vi "cDAQ_VI_Leo_Autotuning.vi"() -> ()   [LabVIEW 2022 SP3]
uses:
  <vilib>/addons/control/pid/autopid.llb/PID autotuning parameters.ctl
  <vilib>/Analysis/baseanly.llb/Mean (DBL).vi
  <vilib>/DAQmx/read.llb/DAQmx Read (Analog 1D Wfm NChan NSamp).vi
  STOP_GLOBAL.vi
  <vilib>/DAQmx/configure/timing.llb/DAQmx Timing (Sample Clock).vi
  <vilib>/addons/control/pid/pid.llb/PID Lead-Lag (DBL).vi
  <vilib>/addons/control/pid/pid.llb/PID Gain Schedule (DBL).vi
  <vilib>/addons/control/pid/pid.llb/PID (DBL).vi
  <vilib>/DAQmx/miscellaneous.llb/DAQmx Fill In Error Info.vi
  <vilib>/Analysis/NI_AALBase.lvlib
  <vilib>/addons/control/pid/NI_PID_pid.lvlib
  <vilib>/ptbypt/NI_PtbyPt.lvlib
  <resource>/objmgr/daqmx.rc
panel:
  out "Inlet Pressure":dynamicdata(graph)
  in  "Channel Array":dbl[](array[slide]) scale=0.0..5.067
  in  "Pressure Scheduling":T1(array[cluster])=[{"PID gains"={"Kc"=7.0, "Ti"=0.001, "Td"=0.0}, "max value"=0.0}] {"max value" format="%.2f"; "PID gains"."Td" format="%#.3g"; "PID gains"."Ti" format="%#.3g"; "PID gains"."Kc" format="%#.3g"}
  out "Runtime Passed?":bool
  in  "RunTime":dbl
  out "Entire Runtime":dbl
  out "Actual Clock Rate":dbl
  out "error out 4":errorcluster
  out "Setpoint profile":dbl
  out "Second Pressure Transducer":cluster{dbl[], dbl[]}(graph)
  out "Second Pressure Transducer":dynamicdata(graph)
  out "Servo Voltage Output":cluster{dbl[], dbl[]}(graph)
  in  "Tab Control":T2(tab)
  out "error out 5":errorcluster
  in  "stop":bool
  in  "Needle Valve Control":dbl[](array[slide]) scale=0.0..1.0
  out "Waveform Chart":cluster{"SP":dbl, dbl}(graph)
  out "Output":dbl(slide) scale=0.0..5.067
  out "Process Variable vs Setpoint":cluster{dbl[], dbl[]}[](graph)
  out "error out":errorcluster
  out "element":dbl
  out "MVT Process variable":dbl
  out "MVT Setpoint":dbl
  in  "SP":dbl format="%.2f"
  out "PID gains out":T3={"proportional gain (Kc)"=1.0, "integral time (Ti, min)"=0.01, "derivative time (Td, min)"=0.0} {"derivative time (Td, min)" format="%.3f"; "integral time (Ti, min)" format="%.3f"; "proportional gain (Kc)" format="%.3f"}
  in  "Insert Gain":bool
  out "output":dbl format="%.2f"
  in  "Autotune":bool
  in  "Reinitialize":bool
  in  "Automatic":bool=TRUE
  in  "Replace Gain":bool
  in  "alpha":dbl=nan format="%.2f"
  out "tuned PID gains":T3={"proportional gain (Kc)"=1.0, "integral time (Ti, min)"=0.01, "derivative time (Td, min)"=0.0} {"derivative time (Td, min)" format="%.3f"; "integral time (Ti, min)" format="%.3f"; "proportional gain (Kc)" format="%.3f"}
  out "Voltage Output":dynamicdata(graph)
  in  "autotuning parameters":T4={"type of controller"=0, "relay cycles"=3, "relay amplitude"=1.0, "control specifications"=2, "PV noise level"=0.1} {"PV noise level" format="%.2f"; "control specifications" items=["normal", "fast", "slow"]; "relay amplitude" format="%.2f"; "type of controller" items=["P", "PI", "PID"]}
  out "index out":i32
  in  "MV:":dbl(slide)=30.8641975308642 scale=0.0..5.067 scale format="%.1f"
  out "Waiting \nfor Start":bool=TRUE
  in  "Start VI":bool
  out "Time":dbl
  in  "Gain Schedule":T1(array[cluster])=[{"PID gains"={"Kc"=7.0, "Ti"=0.001, "Td"=0.0}, "max value"=0.0}] {"max value" format="%.2f"; "PID gains"."Td" format="%#.3g"; "PID gains"."Ti" format="%#.3g"; "PID gains"."Kc" format="%#.3g"}
  out "Steps on Servo":dbl[](array[numeric])
  out "Elapsed Time (s) 2":dbl caption="Elapsed Time (s)"
  out "HAS 3 SECONDS PASSED?":bool
  in  "PRESS TO START":bool
  out "All Channel Graph":cluster{dbl[], dbl[]}[](graph)
  out "Thrust":cluster{dbl[], dbl[]}(graph)
  out "Chamber Pressure":cluster{dbl[], dbl[]}(graph)
  out "Supply Pressure":cluster{dbl[], dbl[]}(graph)
  out "MassFlow":cluster{dbl[], dbl[]}(graph)
  out "Temperature":cluster{dbl[], dbl[]}(graph)
  out "error out 3":errorcluster caption="error out"
  out "error out 2":errorcluster
  in  "rate":dbl=1000.0 format="%0.2f"
  in  "number of samples":i32=100
  in  "File Format":string
  in  "File Name Out":string
  in  "Data Collection Folder":path
  out "Temperature":dynamicdata(graph)
  out "Thrust lb":dynamicdata(graph)
  in  "Types of Testing":enum32{"Test Firing", "Cold Flow Rig"}(tab)
  out "Saving Data":bool
  out "Filename Out":path
  in  "Collect Data?":bool=TRUE caption="Enable"
  in  "Collect Data? 2":bool=TRUE caption="Enable"
  out "Saving Data":bool
  out "Filename Out":path
  out "Supply Pressure PSI":dynamicdata(graph)
  out "Vol Flow L/min":dynamicdata(graph)
  out "Chamber Pressure PSI":dynamicdata(graph)
  # "DATA LOGGING INFORMATION"
  # "Control Loop"
  # "ANALOG VOLTAGE OUTPUT"
  # "RESULTS"
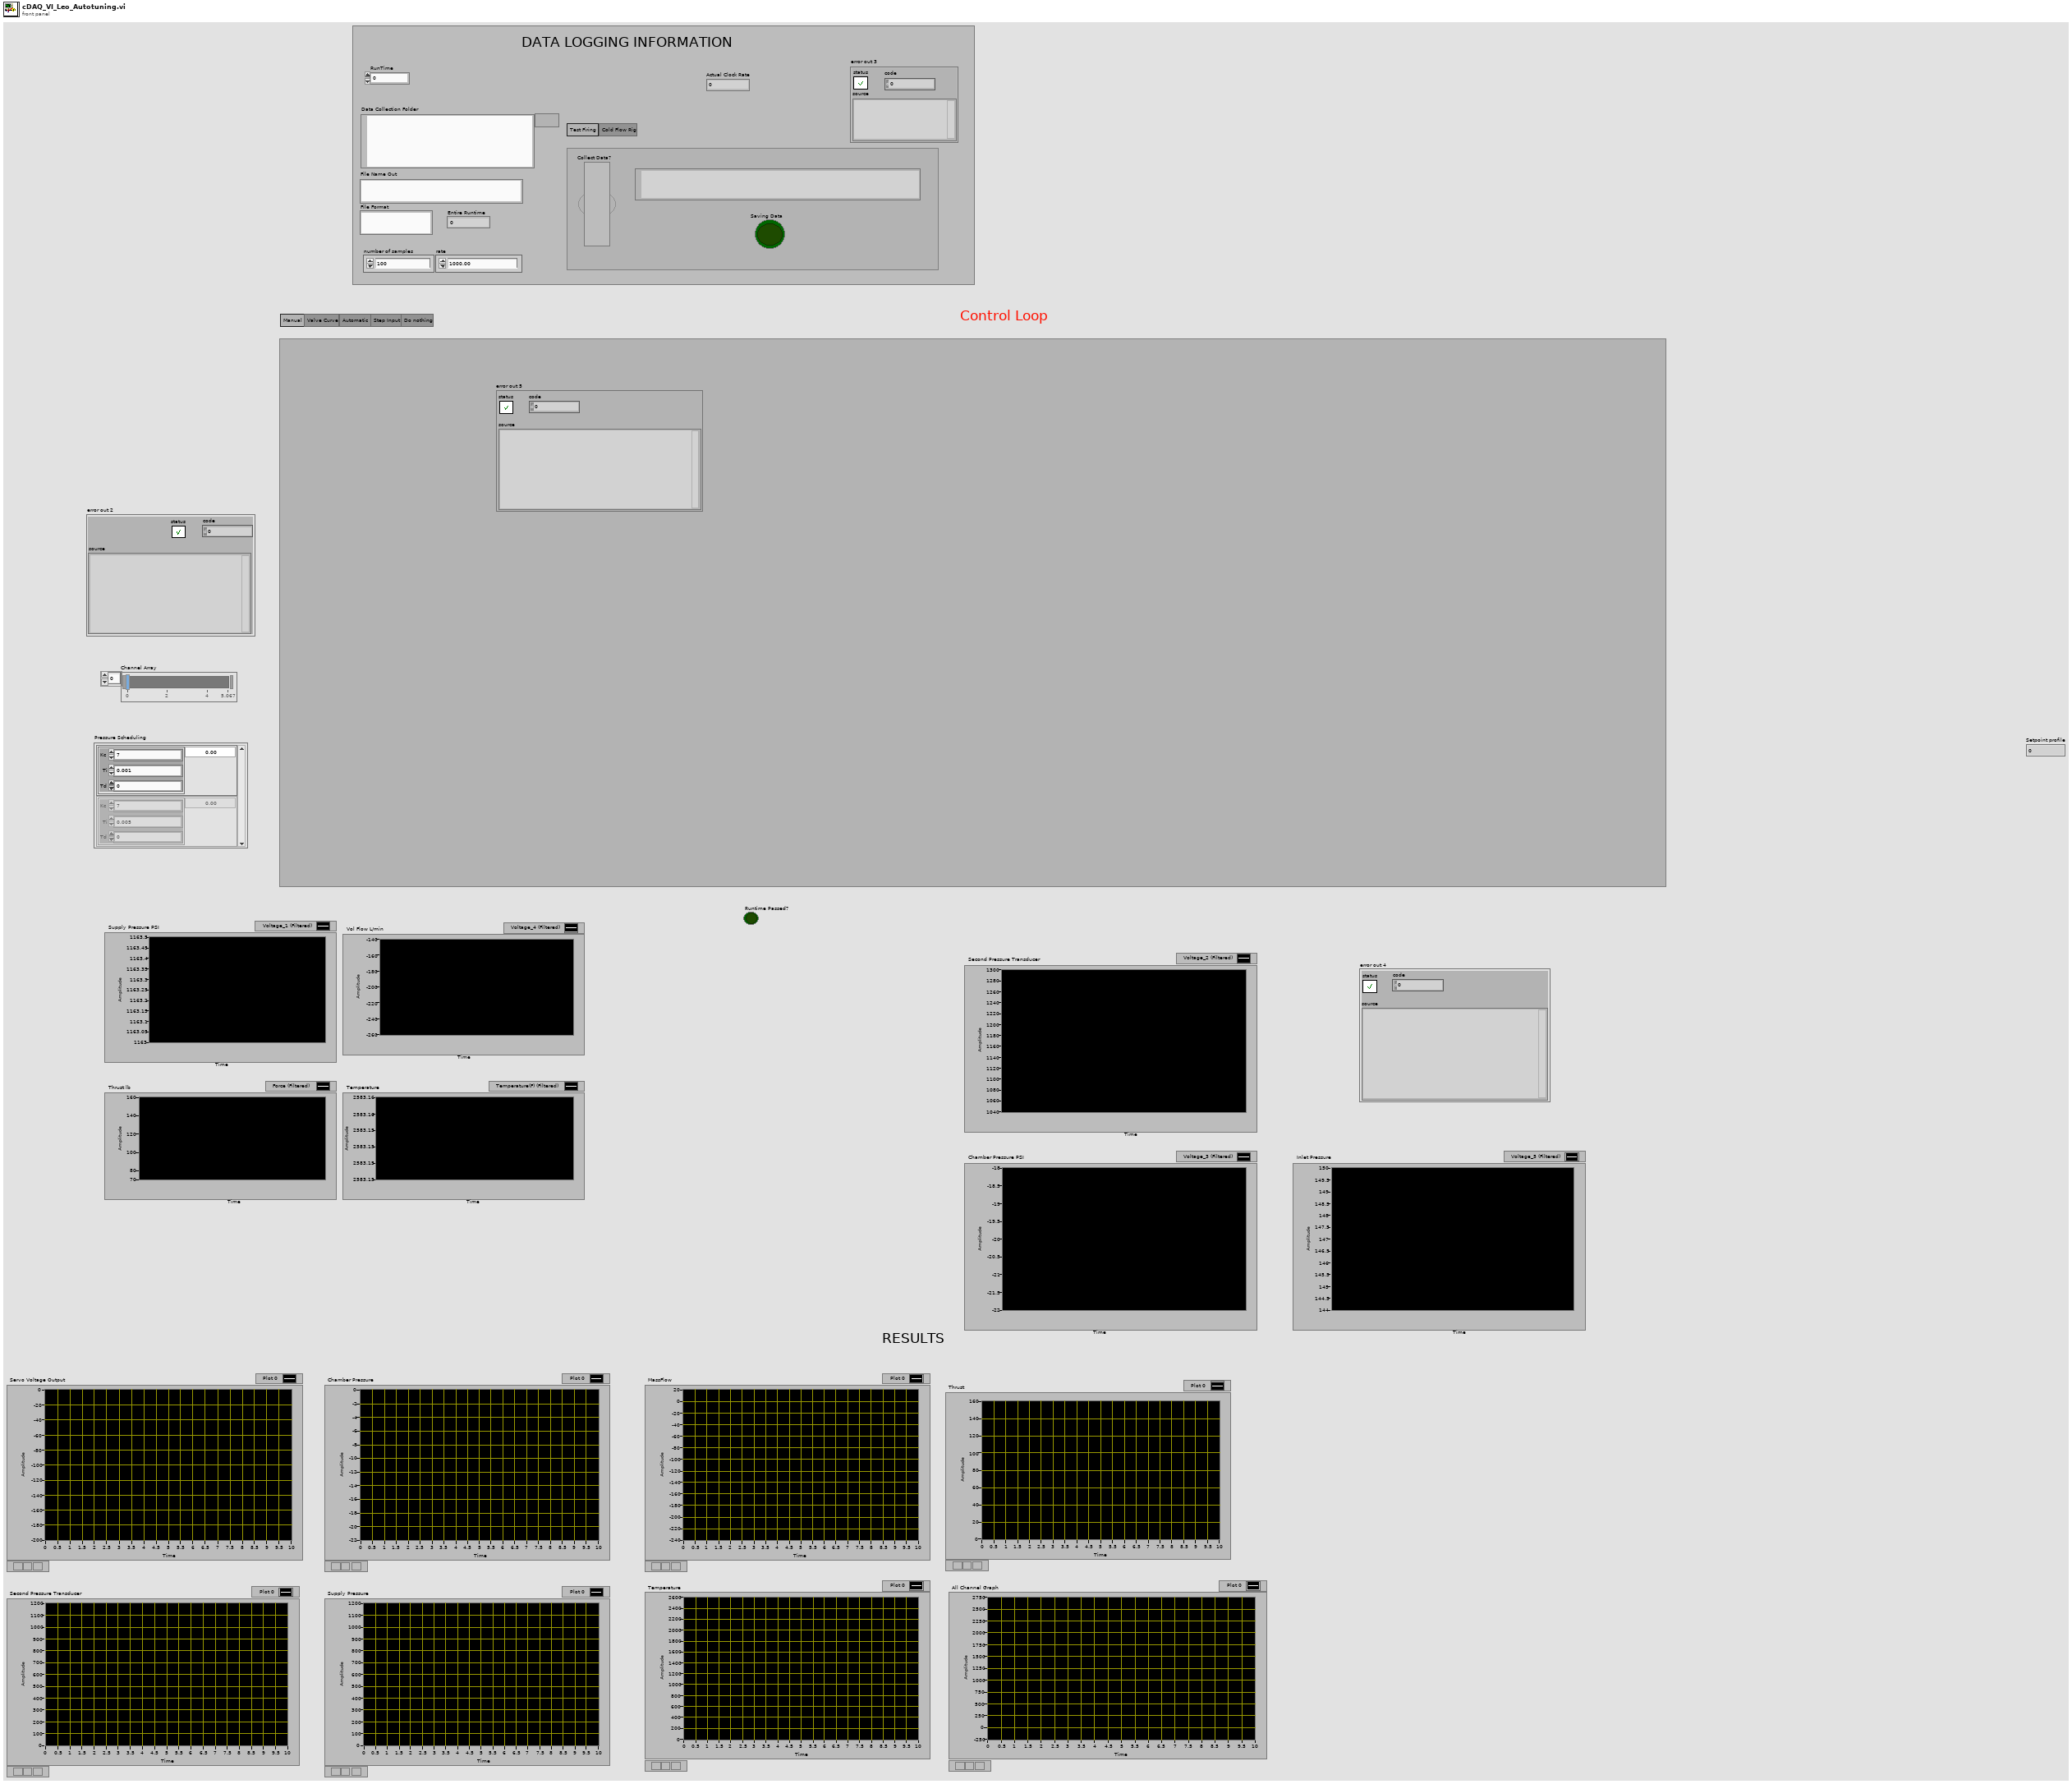
[diagram p1: front panel]
types:
  T1 = cluster{"PID gains":cluster{"Kc":dbl, "Ti":dbl, "Td":dbl}, "max value":dbl}[]
  T2 = enum32{"Manual", "Valve Curve", "Automatic", "Step Input", "Do nothing"}
  T3 = cluster{"proportional gain (Kc)":dbl, "integral time (Ti, min)":dbl, "derivative time (Td, min)":dbl}
  T4 = typedef "PID autotuning parameters.ctl" = cluster{"type of controller":u16, "relay cycles":i32, "relay amplitude":dbl, "control specifications":u16, "PV noise level":dbl}
  T5 = cluster{"Modulus":dbl, "Number of\nComplete Cycles":dbl}
  T6 = cluster{"PID gains":cluster{"Kc":dbl, "Ti":dbl, "Td":dbl}, "max value":dbl}
  T7 = cluster{"Tuned PID gains":cluster{"proportional gain (Kc)":dbl, "integral time (Ti, min)":dbl, "derivative time (Td, min)":dbl}, "MVT Process Variable":dbl}
  T8 = cluster{"Tuned PID gains":cluster{"proportional gain (Kc)":dbl, "integral time (Ti, min)":dbl, "derivative time (Td, min)":dbl}, "max value":dbl}
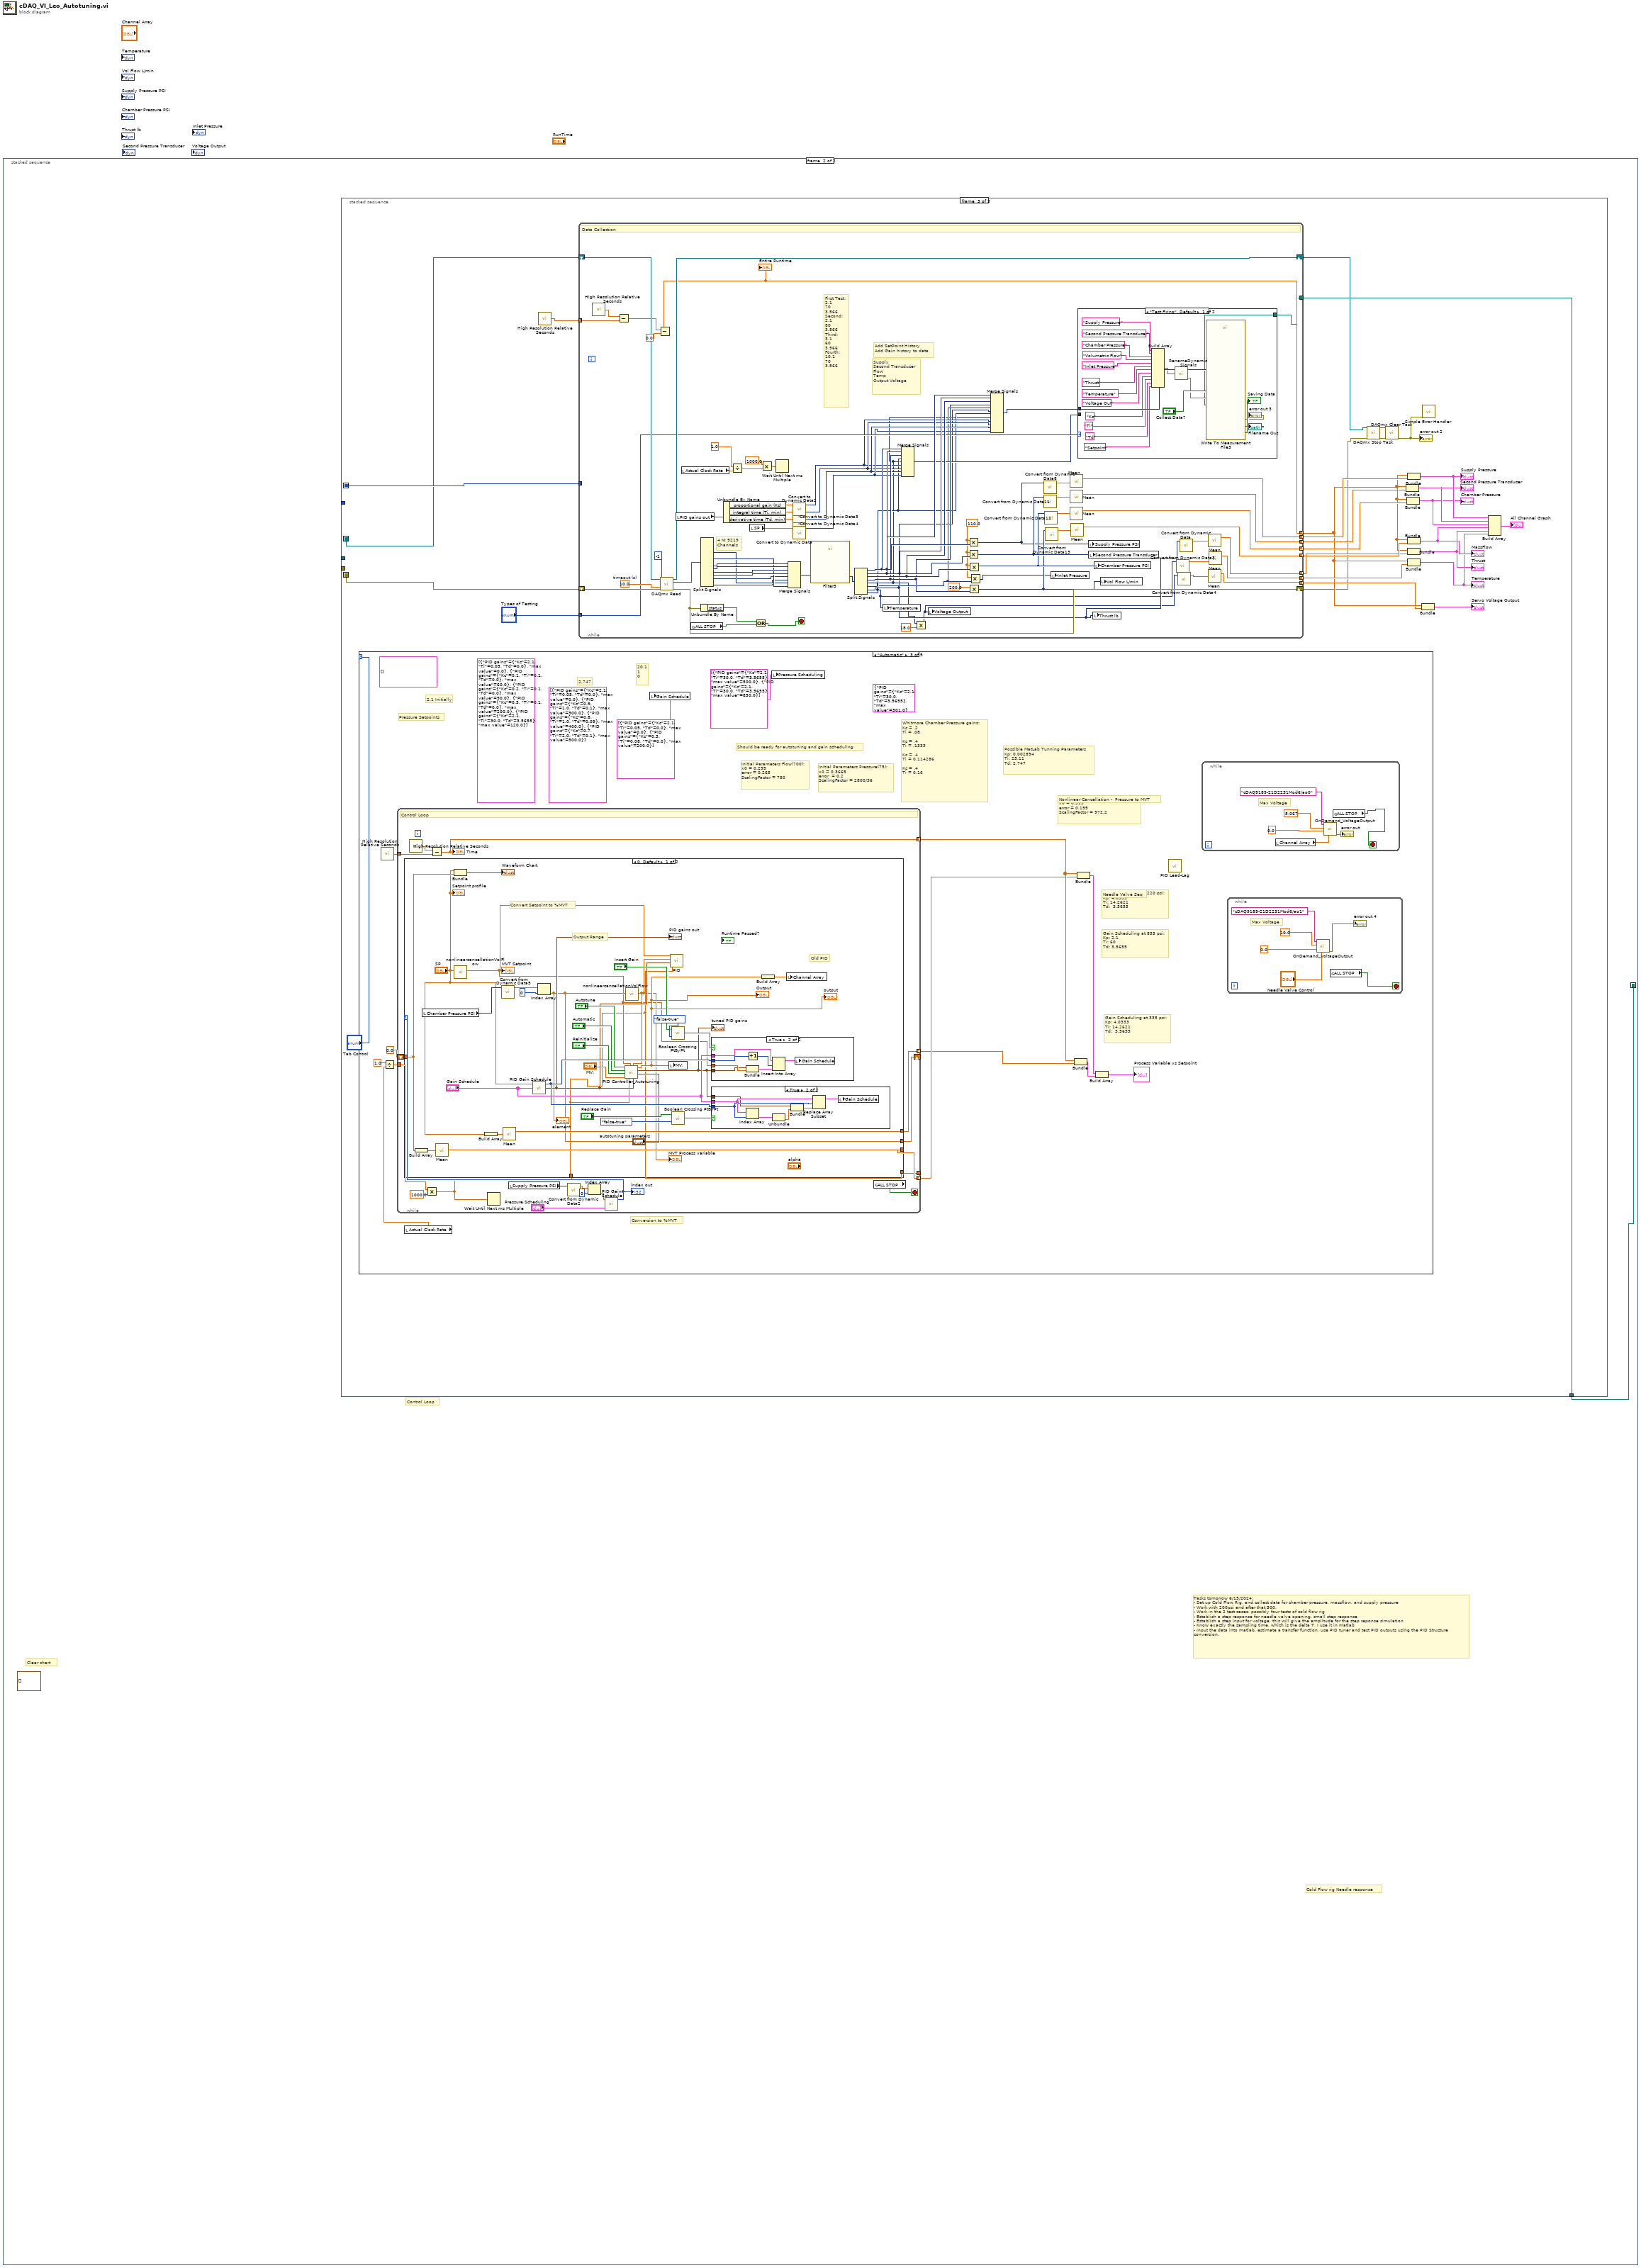
[diagram p0: block diagram]
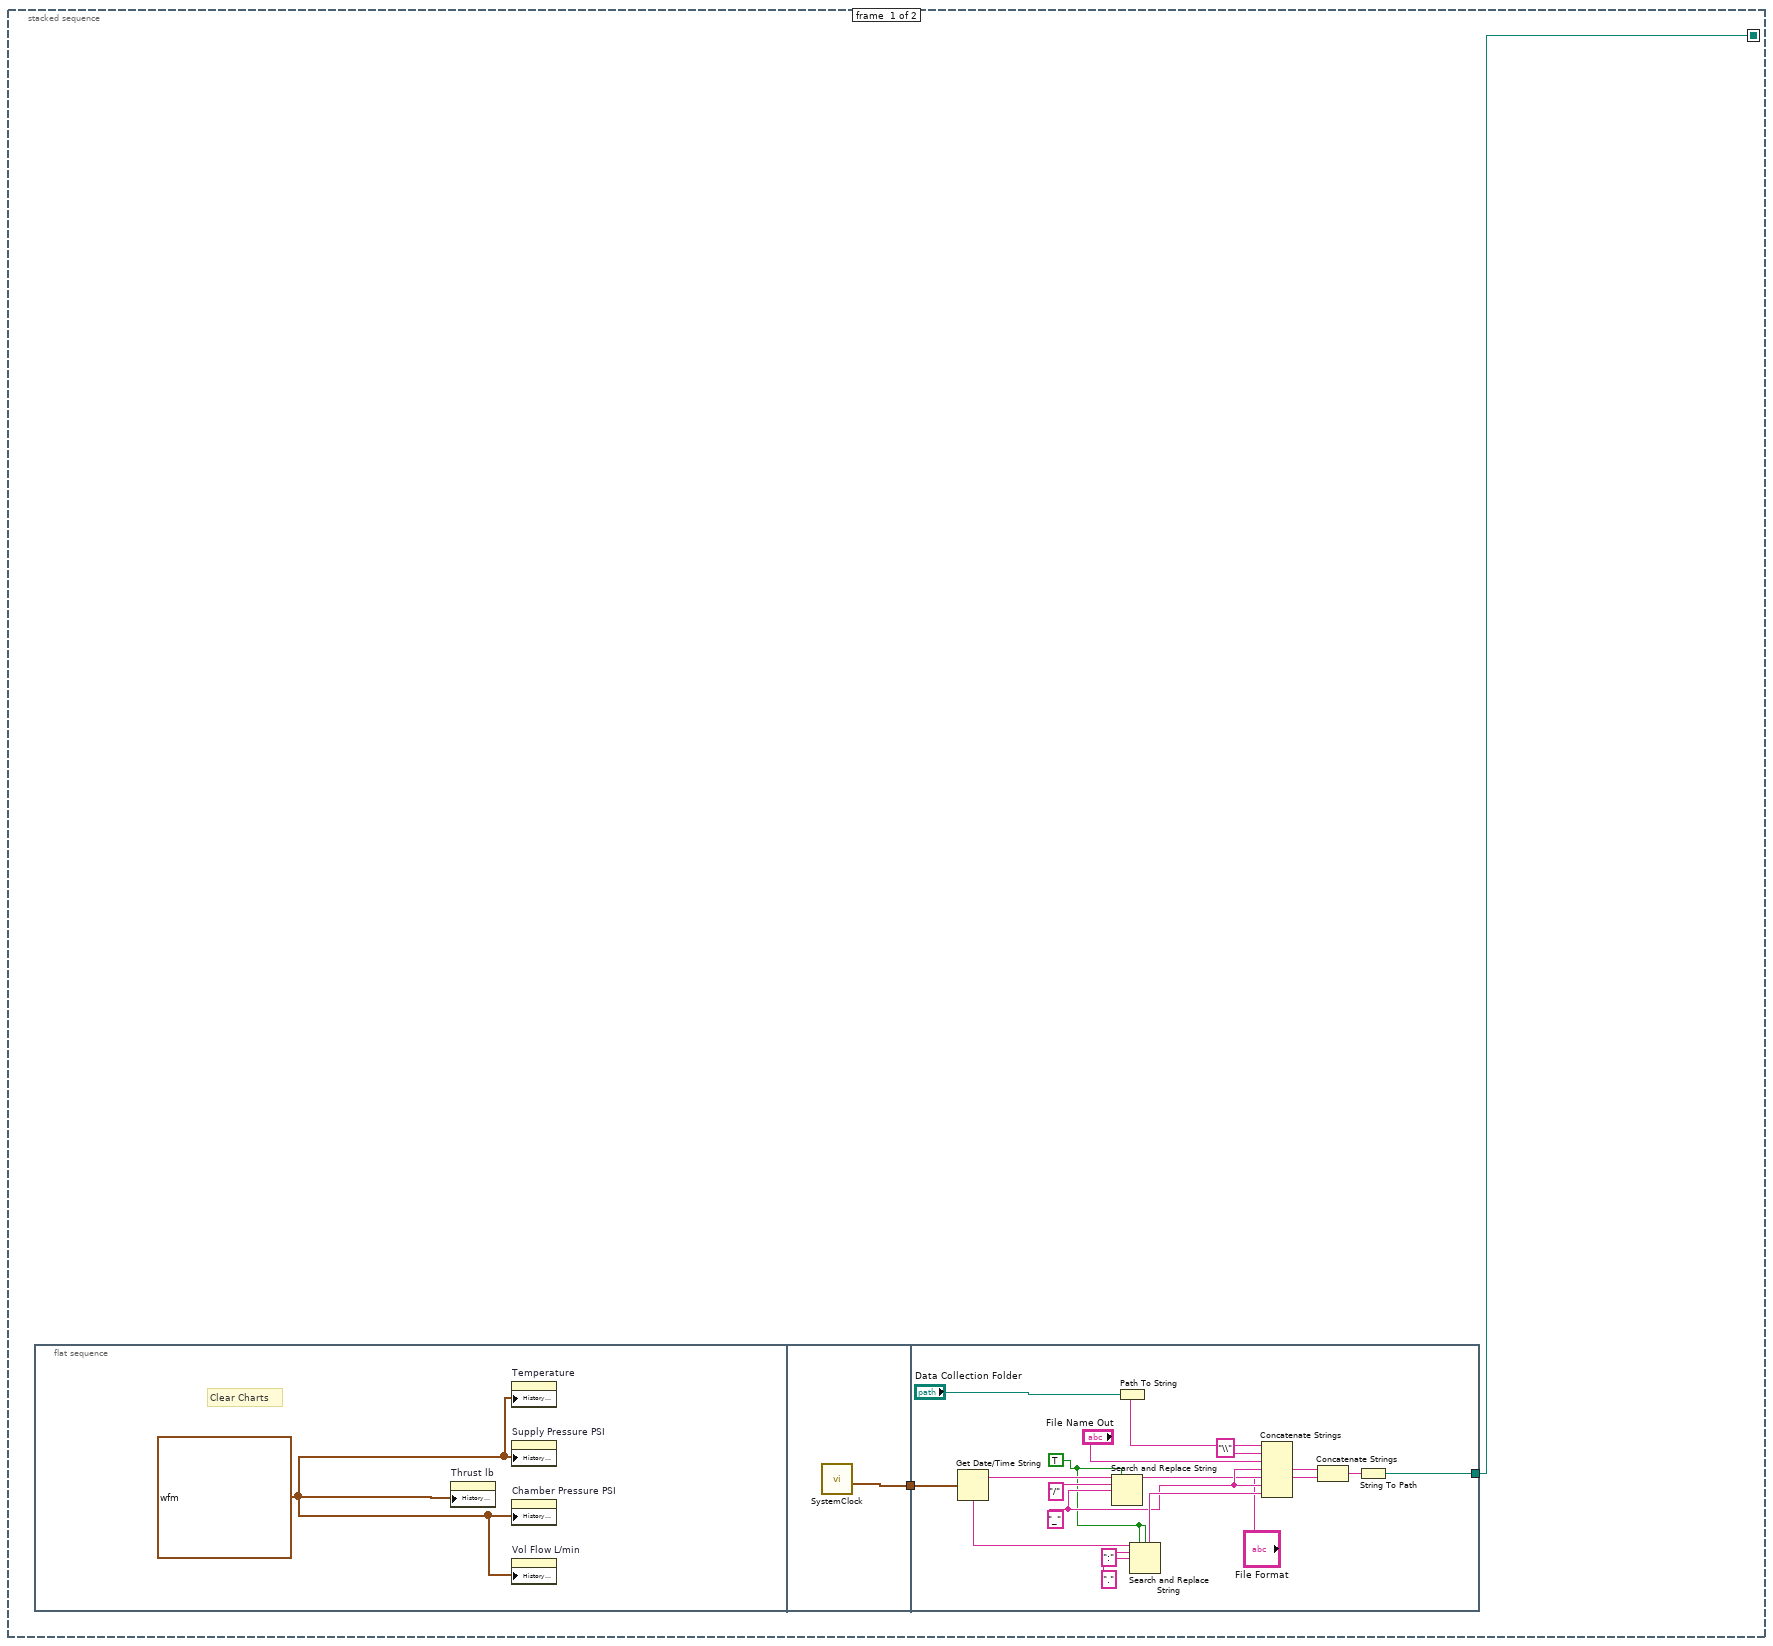
[diagram p2: hidden frame]
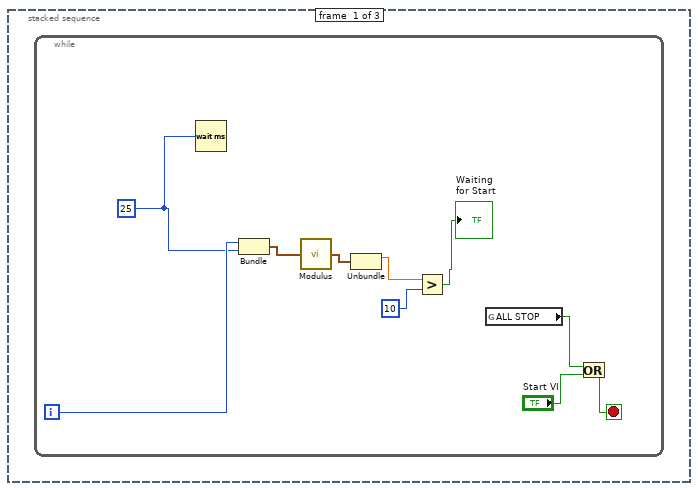
[diagram p3: hidden frame]
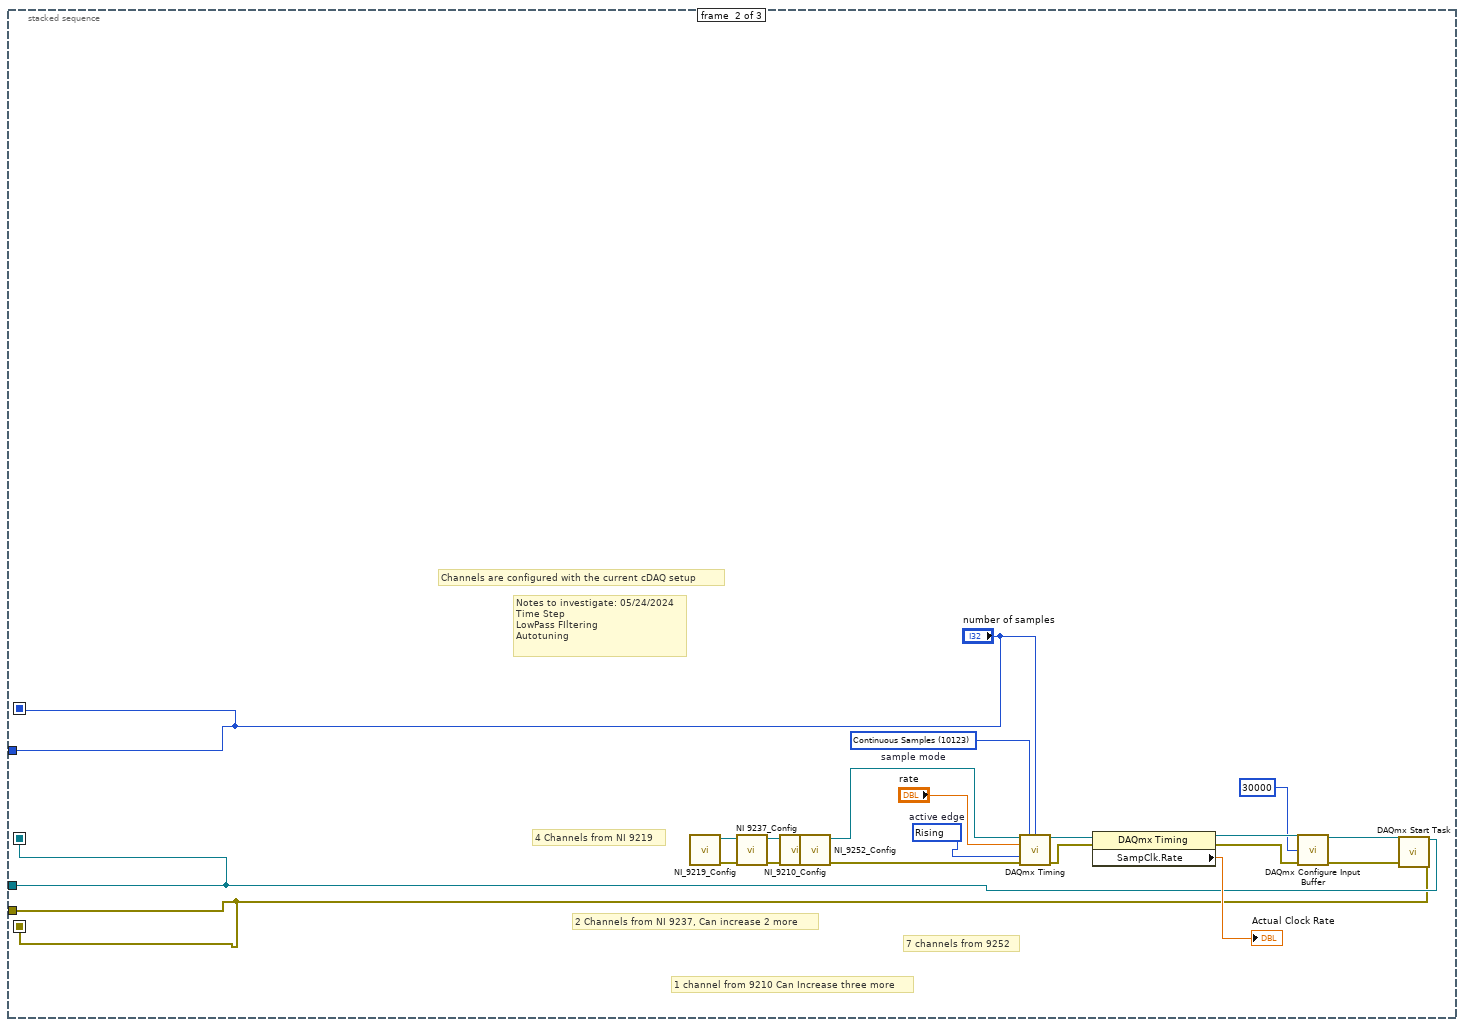
[diagram p4: hidden frame]
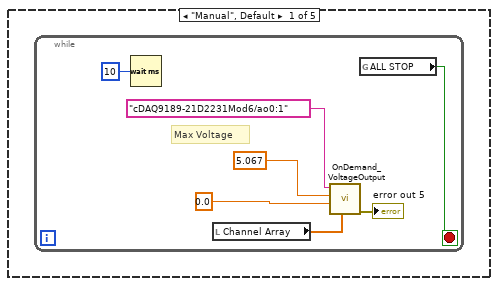
[diagram p5: hidden frame]
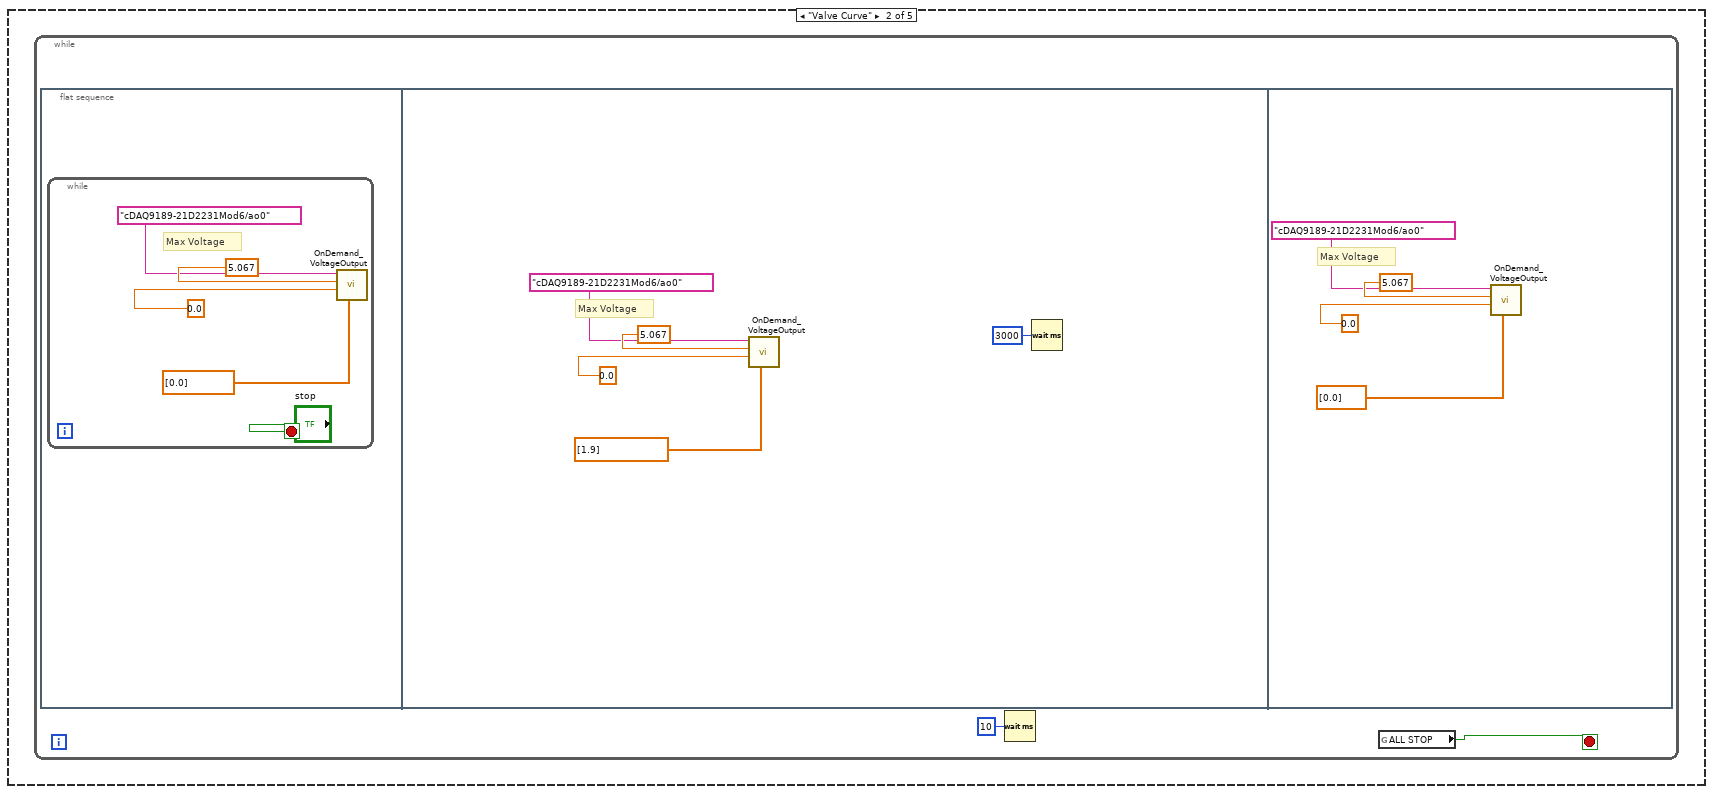
[diagram p6: hidden frame]
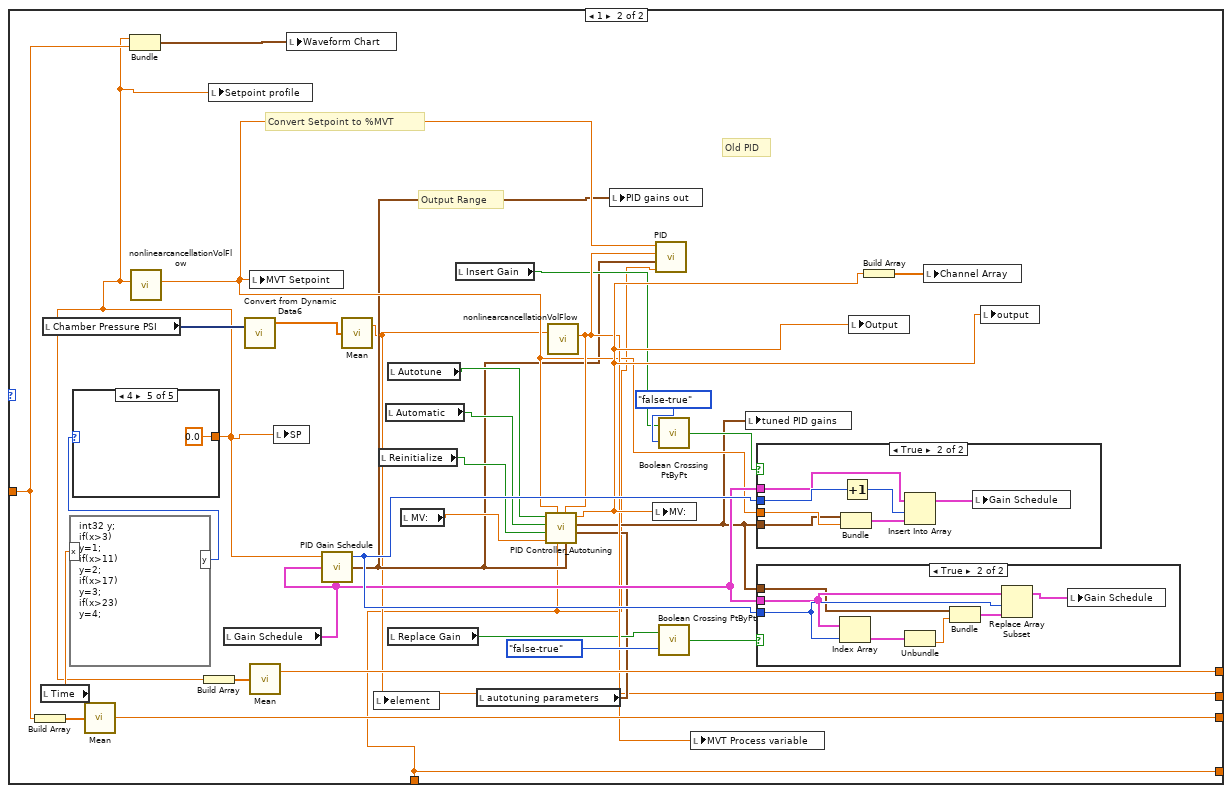
[diagram p9: hidden frame]
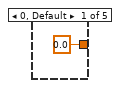
[diagram p10: hidden frame]
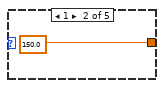
[diagram p11: hidden frame]
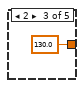
[diagram p12: hidden frame]
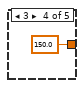
[diagram p13: hidden frame]
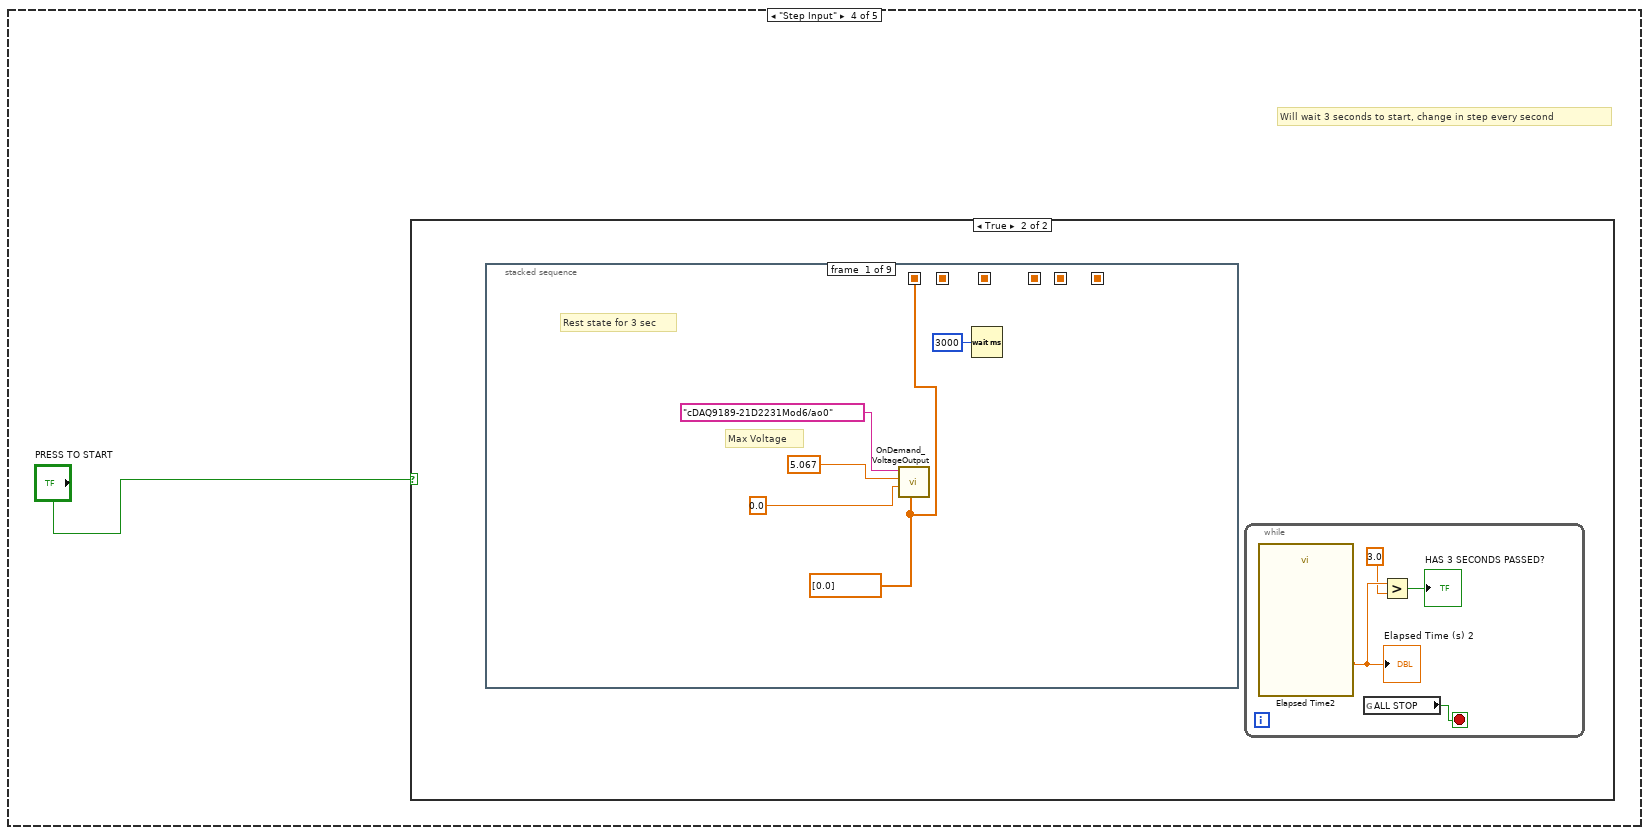
[diagram p16: hidden frame]
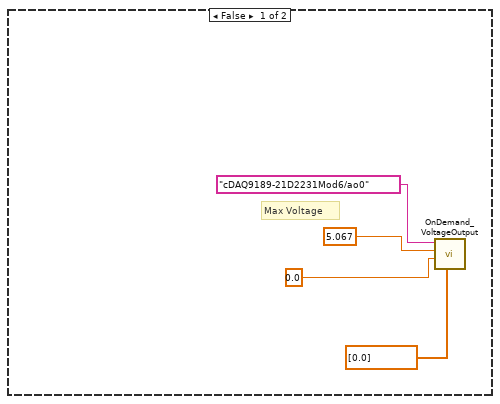
[diagram p17: hidden frame]
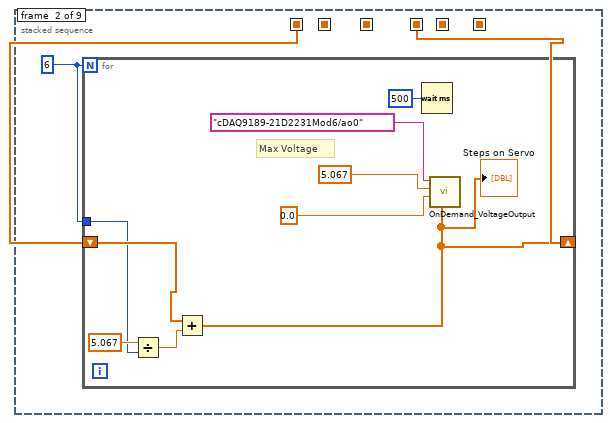
[diagram p18: hidden frame]
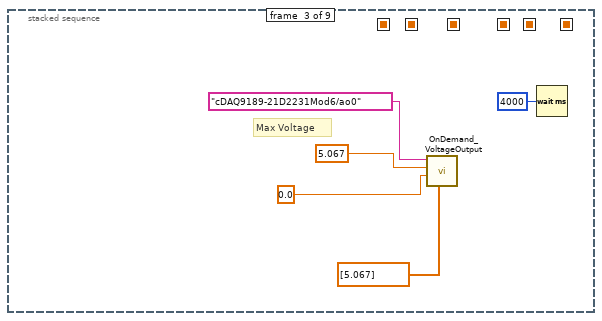
[diagram p19: hidden frame]
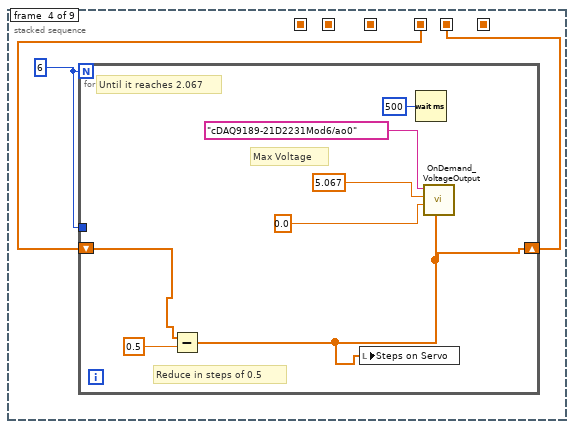
[diagram p20: hidden frame]
diagram:
  n1 = stacked-sequence {
    seq-local: [w1 _] -> [_ w23]
    frame #0 {
      n2 = flat-sequence {
        tunnel: [w4] -> w2
        tunnel: w2 -> [w11]
        tunnel: [w10] -> w1
        frame #0 {
          w3 = waveform(dbl)[] [{"t0"=timestamp(0 s since 1904-01-01), "dt"=1.0, "Y"=[]}]
          # "Clear Charts"
          n3 = property on="Thrust lb" class="WFChart (strict)"("History Data"=w3) -> ()  [unwired: 2 in, 2 out]
          n4 = property on="Temperature" class="WFChart (strict)"("History Data"=w3) -> ()  [unwired: 2 in, 2 out]
          n5 = property on="Supply Pressure PSI" class="WFChart (strict)"("History Data"=w3) -> ()  [unwired: 2 in, 2 out]
          n6 = property on="Chamber Pressure PSI" class="WFChart (strict)"("History Data"=w3) -> ()  [unwired: 2 in, 2 out]
          n7 = property on="Vol Flow L/min" class="WFChart (strict)"("History Data"=w3) -> ()  [unwired: 2 in, 2 out]
        }
        frame #1 {
          n8 = call "SystemClock.vi"() -> ("LabVIEW Time Stamp"=w4:timestamp)  [unwired: 9 in, 2 out]
        }
        frame #2 {
          w6 = TRUE ("replace all? (F)")
          w19 = "_" ("string")
          n9 = Get Date/Time String(seconds (now)=w11) -> (date string=w13:string, time string=w16:string)  [unwired: 2 in]
          n10 = Search and Replace String(replace all?=w6, input string=w13, search string="/", replace string=w19) -> (result string=w15:string)  [unwired: 4 in, 3 out]
          n11 = Path To String(path="Data Collection Folder") -> (string=w8:string)
          n12 = Search and Replace String(replace all?=w6, case sensitive?=w6, input string=w16, search string=":", replace string="." ("replace string (\"\")")) -> (result string=w20:string)  [unwired: 3 in, 3 out]
          n13 = Concatenate Strings(w8, "\\" ("string"), "File Name Out", w19, w15, w19, w20) -> (w21:string)
          n14 = Concatenate Strings(w21, "File Format") -> (w22:string)
          n15 = String To Path(string=w22) -> (path=w10:path)
        }
      }
    }
    frame #1 {
      (unwired) cluster{"setpoint":dbl, dbl}[] [] ("History Data")
      # "Cold Flow rig Needle response"
      # "Tasks tomorrow 6/15/2024:\n- Set up Cold Flow Rig, and collect data for chamber pressure, massflow, and supply pressure\n- Work with 200psi and after that 500.\n- Work in the 2 test cases, possibly four tests of cold flow rig\n- Establish a step response for needle valve opening, small step response\n- Establish a step input for voltage, this will give the amplitude for the step reponse simulation\n- Know exactly the sampling time, which is the delta T, I use it in matlab\n- Input the data into matlab, estimate a transfer function, use PID tuner and test PID outputs using the PID Structure\nconversion."
      # "Control Loop"
      # "Clear chart"
      n16 = stacked-sequence {
        seq-local: [_ "number of samples" _] -> [_ _ w65]
        seq-local: [_ w35 _] -> [_ _ w64]
        seq-local: [_ w34 _] -> [_ _ w63]
        tunnel: w23 -> [_ _ w61]
        tunnel: [_ w35 _] -> _
        tunnel: [_ w34 _] -> _
        tunnel: [_ "number of samples" _] -> _
        frame #0 {
          n17 = while {
            i -> [w33]
            stop <- w25 stop-if-true
            w24 = u32 25 ("milliseconds to wait")
            n18 = Wait (ms)(milliseconds to wait=w24) -> ()  [unwired: 1 out]
            n19 = Bundle(w33, "milliseconds to wait"=w24) -> (w32:cluster{i32, "milliseconds to wait":u32})  [unwired: 1 in]
            n20 = call "Modulus.vi"("Input"=w32) -> ("Output"=w31:T5)
            n21 = Unbundle(w31) -> ("Modulus"=w30:dbl)  [unwired: 1 out]
            n22 = Greater?(x=w30, y=u32 10 ("milliseconds to wait")) -> (0:→"Waiting \nfor Start":bool)
            n23 = global read "STOP_GLOBAL.vi" "ALL STOP"() -> (w27:bool)
            n24 = Or(x=w27, y="Start VI") -> (x .or. y?=w25:bool)
          }
        }
        frame #1 {
          w38 = 10123 items=["Finite Samples"=10178, "Continuous Samples"=10123, "Hardware Timed Single Point"=12522]  # sample mode
          w37 = 10280 items=["Rising"=10280, "Falling"=10171]  # active edge
          # "Notes to investigate: 05/24/2024\nTime Step\nLowPass FIltering\nAutotuning"
          # "Channels are configured with the current cDAQ setup"
          # "7 channels from 9252"
          # "1 channel from 9210 Can Increase three more"
          # "2 Channels from NI 9237, Can increase 2 more"
          # "4 Channels from NI 9219"
          n25 = call "NI_9219_Config.vi"() -> ("error out"=w48:errorcluster, "task out"=w40:refnum<k21>)  [unwired: 10 in]
          n26 = call "NI 9237_Config.vi"("error in"=w48, "task in"=w40) -> ("error out"=w42:errorcluster, "task out"=w41:refnum<k21>)  [unwired: 8 in]
          n27 = call "NI_9210_Config.vi"("error in"=w42, "task in"=w41) -> ("error out"=w44:errorcluster, "task out"=w43:refnum<k21>)  [unwired: 8 in]
          n28 = call "NI_9252_Config.vi"("error in"=w44, "task in"=w43) -> ("error out"=w46:errorcluster, "task out"=w45:refnum<k21>)  [unwired: 8 in]
          n29 = call-poly <vilib>:"DAQmx Timing.vi"("task/channels in"=w45, "sample mode"=w38, "samples per channel"="number of samples", "rate"="rate", "active edge"=w37, "error in"=w46) -> ("task out"=w49:refnum<k21>, "error out"=w50:errorcluster)  [unwired: 8 in]
          n30 = property class="DAQmx Timing"(reference=w49, error in=w50) -> (reference out=w51:refnum<k21>, error out=w52:errorcluster, "SampClk.Rate"=→"Actual Clock Rate":dbl)
          n31 = call <vilib>:"DAQmx Configure Input Buffer.vi"("task/channels in"=w51, "buffer size (in samples per channel)"=u32 30000, "error in"=w52) -> ("task out"=w54:refnum<k21>, "error out"=w53:errorcluster)  [unwired: 11 in]
          n32 = call <vilib>:"DAQmx Start Task.vi"("task/channels in"=w54, "error in"=w53) -> ("task out"=w35:refnum<k21>, "error out"=w34:errorcluster)  [unwired: 12 in]
        }
        frame #2 {
          n33 = case shown="\"Automatic\"" "Tab Control" {
            frame "Manual", Default {
              n34 = while {
                stop <- w90 stop-if-true
                # "Max Voltage"
                n35 = Wait (ms)(milliseconds to wait=u32 10) -> ()  [unwired: 1 out]
                n36 = local read "Channel Array"() -> (w86:dbl[])
                n37 = call "OnDemand_VoltageOutput.vi"("Channel Array"=w86, "minimum voltage"=0.0, "maximum voltage"=5.067, "physical channels"="cDAQ9189-21D2231Mod6/ao0:1") -> ("error out"=→"error out 5":errorcluster)  [unwired: 6 in, 1 out]
                n38 = global read "STOP_GLOBAL.vi" "ALL STOP"() -> (w90:bool)
              }
            }
            frame "Valve Curve" {
              n39 = while {
                stop <- w91 stop-if-true
                n40 = flat-sequence {
                  frame #0 {
                    n41 = while {
                      stop <- "stop" stop-if-true
                      # "Max Voltage"
                      n42 = call "OnDemand_VoltageOutput.vi"("Channel Array"=dbl[] [0.0], "minimum voltage"=0.0, "maximum voltage"=5.067, "physical channels"="cDAQ9189-21D2231Mod6/ao0") -> ()  [unwired: 6 in, 2 out]
                    }
                  }
                  frame #1 {
                    # "Max Voltage"
                    n43 = call "OnDemand_VoltageOutput.vi"("Channel Array"=dbl[] [1.9], "minimum voltage"=0.0, "maximum voltage"=5.067, "physical channels"="cDAQ9189-21D2231Mod6/ao0") -> ()  [unwired: 6 in, 2 out]
                    n44 = Wait (ms)(milliseconds to wait=u32 3000) -> ()  [unwired: 1 out]
                  }
                  frame #2 {
                    # "Max Voltage"
                    n45 = call "OnDemand_VoltageOutput.vi"("Channel Array"=dbl[] [0.0], "minimum voltage"=0.0, "maximum voltage"=5.067, "physical channels"="cDAQ9189-21D2231Mod6/ao0") -> ()  [unwired: 6 in, 2 out]
                  }
                }
                n46 = Wait (ms)(milliseconds to wait=u32 10) -> ()  [unwired: 1 out]
                n47 = global read "STOP_GLOBAL.vi" "ALL STOP"() -> (w91:bool)
              }
            }
            frame "Automatic" {
              (unwired) T6 {"PID gains"={"Kc"=2.1, "Ti"=30.0, "Td"=3.5655}, "max value"=301.0} ("gain schedule")
              (unwired) T1 [{"PID gains"={"Kc"=2.1, "Ti"=0.05, "Td"=0.0}, "max value"=0.0}, {"PID gains"={"Kc"=0.9, "Ti"=1.0, "Td"=0.1}, "max value"=300.0}, {"PID gains"={"Kc"=0.8, "Ti"=1.0, "Td"=0.09}, "max value"=400.0}, {"PID gains"={"Kc"=0.7, "Ti"=2.0, "Td"=0.1}, "max value"=500.0}]
              (unwired) T1 [{"PID gains"={"Kc"=2.1, "Ti"=0.05, "Td"=0.0}, "max value"=0.0}, {"PID gains"={"Kc"=0.1, "Ti"=0.1, "Td"=0.0}, "max value"=60.0}, {"PID gains"={"Kc"=0.2, "Ti"=0.1, "Td"=0.0}, "max value"=90.0}, {"PID gains"={"Kc"=0.5, "Ti"=0.1, "Td"=0.0}, "max value"=200.0}, {"PID gains"={"Kc"=2.1, "Ti"=30.0, "Td"=3.5655}, "max value"=120.0}] ("PID gain schedule 2")
              (unwired) T1 [] ("PID gain schedule 2")
              # "Whitmore Chamber Pressure gains:\nKc = .2\nTi = .08\n\nKc = .4\nTi = .1333\n\nKc = .4\nTi = 0.114286\n\nKc = .4\nTi = 0.16"
              # "Conversion to %MVT"
              # "Pressure Setpoints"
              # "Initial Parameters Pressure(75):\nx0 = 0.3665\nerror  = 0.2\nScalingFactor = 2800/36"
              # "Initial Parameters Flow(700):\nx0 = 0.295\nerror = 0.265\nScalingFactor = 780"
              # "2.1 Initially"
              # "20.1\n1\n0"
              # "2.747"
              # "Should be ready for autotuning and gain scheduling"
              # "Possible parameters for 800 SLM:\nx0 = 0.315\nerror = 0.195\nScalingFactor = 972.2"
              # "Nonlinear Cancellation -  Pressure to MVT"
              # "Possible MatLab Tunning Parameters\nKp: 0.002894\nTi: 25.11\nTd: 2.747"
              # "Gain Scheduling at 335 psi:\nKp: 4.0333\nTi: 14.2621\nTd:  3.5655"
              # "Gain Scheduling at 855 psi:\nKp: 2.1\nTi: 60\nTd: 3.5655"
              # "Gain Scheduling at 220 psi:\nKp: 4.0333\nTi: 14.2621\nTd:  3.5655"
              # "Needle Valve Seq"
              n48 = call <vilib>:"High Resolution Relative Seconds.vi"() -> ("relative seconds"=w114:dbl)
              n49 = local read "Actual Clock Rate"() -> (w113:dbl)
              n50 = Divide(x=1.0, y=w113) -> (x/y=w111:dbl)
              n51 = while {
                shift-right: [w143] -> _
                shift-left: 0.0 -> [w141]
                tunnel: [w142] -> w117 mode=indexing
                tunnel: [w149] -> w110 mode=indexing
                tunnel: [w148] -> w109 mode=indexing
                tunnel: w114 -> [w147]
                tunnel: [w144] -> _
                tunnel: w111 -> [w133]
                stop <- w145 stop-if-true
                # "Control Loop"
                n52 = call <vilib>:"High Resolution Relative Seconds.vi"() -> ("relative seconds"=w146:dbl)
                n53 = Multiply(x=w133, y=1000.0) -> (x*y=w132:dbl)
                n54 = Subtract(x=w146, y=w147) -> (x-y=w142:dbl)
                "Time" <- w142
                n55 = Wait Until Next ms Multiple(millisecond multiple=w132) -> ()  [unwired: 1 out]
                n56 = local read "Supply Pressure PSI"() -> (w140:dynamicdata)
                n57 = call "Convert from Dynamic Data2"("Dynamic Data Type"=w140) -> ("Array"=w139:dbl[])  [unwired: 3 in]
                n58 = Index Array(array=w139, index=0) -> (element=w138:dbl)
                n59 = call-poly <vilib>:"PID Gain Schedule.vi"("PID gain schedule"="Pressure Scheduling", "gain scheduling value"=w138) -> ("index out"=w135:i32)  [unwired: 2 in, 1 out]
                "index out" <- w135
                n60 = case shown="0, Default" w135 {
                  tunnel: [w180 w226] -> w149
                  tunnel: [w179 w225] -> w148
                  tunnel: [w151 w200] -> w144
                  tunnel: [w158 w201] -> w143
                  tunnel: w141 -> [w155 w216]
                  tunnel: w132 -> [w151 w200]
                  frame 0, Default {
                    # "Old PID"
                    # "Convert Setpoint to %MVT"
                    # "Output Range"
                    n61 = Build Array(w155) -> (w154:dbl[])
                    n62 = local read "Chamber Pressure PSI"() -> (w166:dynamicdata)
                    n63 = call-poly <vilib>:"Mean.vi"("X"=w154) -> ("mean"=w180:dbl)  [unwired: 1 out]
                    n64 = Bundle("SP"="SP", w155) -> (→"Waveform Chart":cluster{"SP":dbl, dbl})  [unwired: 1 in]
                    n65 = call "nonlinearcancellationVolFlow.vi"("input variable"="SP") -> ("MVT Process Variable"=w153:dbl)  [unwired: 10 in]
                    "MVT Setpoint" <- w153
                    n66 = Build Array("SP") -> (w177:dbl[])
                    n67 = call "Convert from Dynamic Data5"("Dynamic Data Type"=w166) -> ("Array"=w176:dbl[])  [unwired: 3 in]
                    n68 = call-poly <vilib>:"Mean.vi"("X"=w177) -> ("mean"=w179:dbl)  [unwired: 1 out]
                    n69 = call-poly <vilib>:"PID Gain Schedule.vi"("PID gain schedule"="Gain Schedule", "gain scheduling value"="SP") -> ("PID gains out"=w161:T3, "index out"=w169:i32)  [unwired: 2 in]
                    "PID gains out" <- w161
                    n70 = Index Array(array=w176, index=0) -> (element=w158:dbl)
                    "element" <- w158
                    n71 = call "nonlinearcancellationVolFlow.vi"("input variable"=w158) -> ("MVT Process Variable"=w156:dbl)  [unwired: 10 in]
                    "MVT Process variable" <- w156
                    n72 = call "PID Controller_Autotuning.vi"("autotuning parameters"="autotuning parameters", "PID gains in"=w161, "process variable"=w156, "dt (s)"=w151, "setpoint"=w153, "manipulated variable"="MV:", "Reinitialize"="Reinitialize", "Automatic"="Automatic", "Autotune"="Autotune") -> ("Tuned PID gains"=w157:T3, "output"=w159:dbl)  [unwired: 1 in]
                    "tuned PID gains" <- w157
                    "Output" <- w159
                    "output" <- w159
                    n73 = local write "MV:"(w159) -> ()
                    n74 = call-poly <vilib>:"PID.vi"("dt (s)"=w151, "PID gains"=w161, "process variable"=w156, "setpoint"=w153) -> ()  [unwired: 6 in, 2 out]
                    n75 = call <vilib>:"Boolean Crossing PtByPt.vi"("direction"=enum16{"either", "false-true", "true-false"}."false-true", "input"="Insert Gain") -> ("crossing"=w174:bool)  [unwired: 1 in]
                    n76 = call <vilib>:"Boolean Crossing PtByPt.vi"("direction"=enum16{"either", "false-true", "true-false"}."false-true", "input"="Replace Gain") -> ("crossing"=w170:bool)  [unwired: 1 in]
                    n77 = case shown="True" w174 {
                      tunnel: w169 -> [_ w194]
                      tunnel: "Gain Schedule" -> [_ w192]
                      tunnel: w153 -> [_ w191]
                      tunnel: w157 -> [_ w189]
                      frame False {
                      }
                      frame True {
                        n78 = Bundle("Tuned PID gains"=w189, "MVT Process Variable"=w191) -> (w188:T7)  [unwired: 1 in]
                        n79 = Increment(x=w194) -> (x+1=w193:i32)
                        n80 = Insert Into Array(array=w192, index=w193, new element=w188) -> (w190:T1)
                        n81 = local write "Gain Schedule"(w190) -> ()
                      }
                    }
                    n82 = case shown="True" w170 {
                      tunnel: w169 -> [_ w185]
                      tunnel: "Gain Schedule" -> [_ w184]
                      tunnel: w157 -> [_ w182]
                      frame False {
                      }
                      frame True {
                        n83 = Index Array(array=w184, index=w185) -> (element=w187:T6)
                        n84 = Unbundle(w187) -> ("max value"=w186:dbl)  [unwired: 1 out]
                        n85 = Bundle("Tuned PID gains"=w182, "max value"=w186) -> (w181:T8)  [unwired: 1 in]
                        n86 = Replace Array Subset(array=w184, new element=w181, index=w185) -> (w183:T1)
                        n87 = local write "Gain Schedule"(w183) -> ()
                      }
                    }
                    n88 = Build Array(w159) -> (w150:dbl[])
                    n89 = local write "Channel Array"(w150) -> ()
                    "Setpoint profile" <- "SP"
                  }
                  frame 1 {
                    # "Old PID"
                    # "Convert Setpoint to %MVT"
                    # "Output Range"
                    n90 = Build Array(w216) -> (w215:dbl[])
                    n91 = local read "Time"() -> (w198:dbl)
                    n92 = local read "Chamber Pressure PSI"() -> (w218:dynamicdata)
                    n93 = formula code="int32 y;\nif(x>3)\ny=1;\nif(x>11)\ny=2;\nif(x>17)\ny=3;\nif(x>23)\ny=4;"("x"=w198) -> ("y"=w199:i32)
                    n94 = case shown="4" w199 {
                      tunnel: [0.0 ("SP") 150.0 ("SP") 130.0 ("SP") 150.0 ("SP") 0.0 ("SP")] -> w196
                      frame 0, Default {
                      }
                      frame 1 {
                      }
                      frame 2 {
                      }
                      frame 3 {
                      }
                      frame 4 {
                      }
                    }
                    n95 = call-poly <vilib>:"Mean.vi"("X"=w215) -> ("mean"=w226:dbl)  [unwired: 1 out]
                    n96 = Bundle("SP"=w196, w216) -> (w208:cluster{"SP":dbl, dbl})  [unwired: 1 in]
                    n97 = call "nonlinearcancellationVolFlow.vi"("input variable"=w196) -> ("MVT Process Variable"=w206:dbl)  [unwired: 10 in]
                    n98 = Build Array(w196) -> (w224:dbl[])
                    n99 = local write "Setpoint profile"(w196) -> ()
                    n100 = local read "Gain Schedule"() -> (w214:T1)
                    n101 = call "Convert from Dynamic Data6"("Dynamic Data Type"=w218) -> ("Array"=w197:dbl[])  [unwired: 3 in]
                    n102 = local write "MVT Setpoint"(w206) -> ()
                    n103 = call-poly <vilib>:"Mean.vi"("X"=w224) -> ("mean"=w225:dbl)  [unwired: 1 out]
                    n104 = local write "SP"(w196) -> ()
                    n105 = local write "Waveform Chart"(w208) -> ()
                    n106 = call-poly <vilib>:"PID Gain Schedule.vi"("PID gain schedule"=w214, "gain scheduling value"=w196) -> ("PID gains out"=w205:T3, "index out"=w219:i32)  [unwired: 2 in]
                    n107 = call-poly <vilib>:"Mean.vi"("X"=w197) -> ("mean"=w201:dbl)  [unwired: 1 out]
                    n108 = local write "element"(w201) -> ()
                    n109 = local read "Reinitialize"() -> (w211:bool)
                    n110 = local read "Automatic"() -> (w212:bool)
                    n111 = local read "Autotune"() -> (w213:bool)
                    n112 = local read "Replace Gain"() -> (w204:bool)
                    n113 = local read "MV:"() -> (w210:dbl)
                    n114 = local read "Insert Gain"() -> (w207:bool)
                    n115 = local read "autotuning parameters"() -> (w202:T4)
                    n116 = call "nonlinearcancellationVolFlow.vi"("input variable"=w201) -> ("MVT Process Variable"=w209:dbl)  [unwired: 10 in]
                    n117 = call "PID Controller_Autotuning.vi"("autotuning parameters"=w202, "PID gains in"=w205, "process variable"=w209, "dt (s)"=w200, "setpoint"=w206, "manipulated variable"=w210, "Reinitialize"=w211, "Automatic"=w212, "Autotune"=w213) -> ("Tuned PID gains"=w203:T3, "output"=w217:dbl)  [unwired: 1 in]
                    n118 = local write "PID gains out"(w205) -> ()
                    n119 = local write "MV:"(w217) -> ()
                    n120 = call-poly <vilib>:"PID.vi"("dt (s)"=w200, "PID gains"=w205, "process variable"=w209, "setpoint"=w206) -> ()  [unwired: 6 in, 2 out]
                    n121 = call <vilib>:"Boolean Crossing PtByPt.vi"("direction"=enum16{"either", "false-true", "true-false"}."false-true", "input"=w207) -> ("crossing"=w222:bool)  [unwired: 1 in]
                    n122 = call <vilib>:"Boolean Crossing PtByPt.vi"("direction"=enum16{"either", "false-true", "true-false"}."false-true", "input"=w204) -> ("crossing"=w220:bool)  [unwired: 1 in]
                    n123 = local write "MVT Process variable"(w209) -> ()
                    n124 = local write "tuned PID gains"(w203) -> ()
                    n125 = case shown="True" w222 {
                      tunnel: w219 -> [_ w245]
                      tunnel: w214 -> [_ w243]
                      tunnel: w206 -> [_ w242]
                      tunnel: w203 -> [_ w241]
                      frame False {
                      }
                      frame True {
                        n126 = Bundle("Tuned PID gains"=w241, "MVT Process Variable"=w242) -> (w240:T7)  [unwired: 1 in]
                        n127 = Increment(x=w245) -> (x+1=w244:i32)
                        n128 = Insert Into Array(array=w243, index=w244, new element=w240) -> (w239:T1)
                        n129 = local write "Gain Schedule"(w239) -> ()
                      }
                    }
                    n130 = case shown="True" w220 {
                      tunnel: w219 -> [_ w236]
                      tunnel: w214 -> [_ w235]
                      tunnel: w203 -> [_ w234]
                      frame False {
                      }
                      frame True {
                        n131 = Index Array(array=w235, index=w236) -> (element=w238:T6)
                        n132 = Unbundle(w238) -> ("max value"=w237:dbl)  [unwired: 1 out]
                        n133 = Bundle("Tuned PID gains"=w234, "max value"=w237) -> (w233:T8)  [unwired: 1 in]
                        n134 = Replace Array Subset(array=w235, new element=w233, index=w236) -> (w232:T1)
                        n135 = local write "Gain Schedule"(w232) -> ()
                      }
                    }
                    n136 = local write "Output"(w217) -> ()
                    n137 = Build Array(w217) -> (w195:dbl[])
                    n138 = local write "Channel Array"(w195) -> ()
                    n139 = local write "output"(w217) -> ()
                  }
                }
                n140 = global read "STOP_GLOBAL.vi" "ALL STOP"() -> (w145:bool)
              }
              n141 = local write "Gain Schedule"(T1 [{"PID gains"={"Kc"=2.1, "Ti"=0.05, "Td"=0.0}, "max value"=0.0}, {"PID gains"={"Kc"=0.3, "Ti"=0.08, "Td"=0.0}, "max value"=200.0}]) -> ()
              n142 = local write "Pressure Scheduling"(T1 [{"PID gains"={"Kc"=2.1, "Ti"=30.0, "Td"=3.5655}, "max value"=500.0}, {"PID gains"={"Kc"=2.1, "Ti"=30.0, "Td"=3.5655}, "max value"=850.0}]) -> ()
              n143 = Bundle(w117, w109) -> (w118:cluster{dbl[], dbl[]})  [unwired: 1 in]
              n144 = Bundle(w117, w110) -> (w115:cluster{dbl[], dbl[]})  [unwired: 1 in]
              n145 = Build Array(w115, w118) -> (→"Process Variable vs Setpoint":cluster{dbl[], dbl[]}[])
              n146 = call-poly <vilib>:"PID Lead-Lag.vi"() -> ()  [unwired: 8 in, 2 out]
              n147 = while {
                stop <- w126 stop-if-true
                # "Max Voltage"
                n148 = local read "Channel Array"() -> (w129:dbl[])
                n149 = call "OnDemand_VoltageOutput.vi"("Channel Array"=w129, "minimum voltage"=0.0, "maximum voltage"=5.067, "physical channels"="cDAQ9189-21D2231Mod6/ao0") -> ("error out"=→"error out":errorcluster)  [unwired: 6 in, 1 out]
                n150 = global read "STOP_GLOBAL.vi" "ALL STOP"() -> (w126:bool)
              }
              n151 = while {
                stop <- w125 stop-if-true
                # "Max Voltage"
                n152 = call "OnDemand_VoltageOutput.vi"("Channel Array"="Needle Valve Control", "minimum voltage"=0.0, "maximum voltage"=10.0, "physical channels"="cDAQ9189-21D2231Mod6/ao1") -> ("error out"=→"error out 4":errorcluster)  [unwired: 6 in, 1 out]
                n153 = global read "STOP_GLOBAL.vi" "ALL STOP"() -> (w125:bool)
              }
            }
            frame "Step Input" {
              # "Will wait 3 seconds to start, change in step every second"
              n154 = case shown="True" "PRESS TO START" {
                frame False {
                  # "Max Voltage"
                  n155 = call "OnDemand_VoltageOutput.vi"("Channel Array"=dbl[] [0.0], "minimum voltage"=0.0, "maximum voltage"=5.067, "physical channels"="cDAQ9189-21D2231Mod6/ao0") -> ()  [unwired: 6 in, 2 out]
                }
                frame True {
                  n156 = stacked-sequence {
                    seq-local: [_ _ _ _ _ w298 _ _ _] -> [_ _ _ _ _ _ w308 _ _]
                    seq-local: [_ _ _ _ _ _ w307 _ _] -> [_ _ _ _ _ _ _ w317 _]
                    seq-local: [w255 _ _ _ _ _ _ _ _] -> [_ w261 _ _ _ _ _ _ _]
                    seq-local: [_ w260 _ _ _ _ _ _ _] -> [_ _ _ w278 _ _ _ _ _]
                    seq-local: [_ _ _ w277 _ _ _ _ _] -> [_ _ _ _ w288 _ _ _ _]
                    seq-local: [_ _ _ _ w287 _ _ _ _] -> [_ _ _ _ _ w297 _ _ _]
                    frame #0 {
                      w255 = dbl[] [0.0]
                      # "Rest state for 3 sec"
                      # "Max Voltage"
                      n157 = call "OnDemand_VoltageOutput.vi"("Channel Array"=w255, "minimum voltage"=0.0, "maximum voltage"=5.067, "physical channels"="cDAQ9189-21D2231Mod6/ao0") -> ()  [unwired: 6 in, 2 out]
                      n158 = Wait (ms)(milliseconds to wait=u32 3000) -> ()  [unwired: 1 out]
                    }
                    frame #1 {
                      w262 = 6
                      n159 = for {
                        N: w262 -> [_]
                        shift-right: [w263] -> w260
                        shift-left: w261 -> [w270]
                        tunnel: w262 -> [w264]
                        # "Max Voltage"
                        n160 = Divide(x=5.067, y=w264) -> (x/y=w266:dbl)
                        n161 = Add(x=w270, y=w266) -> (x+y=w263:dbl[])
                        "Steps on Servo" <- w263
                        n162 = Wait (ms)(milliseconds to wait=u32 500) -> ()  [unwired: 1 out]
                        n163 = call "OnDemand_VoltageOutput.vi"("Channel Array"=w263, "minimum voltage"=0.0, "maximum voltage"=5.067, "physical channels"="cDAQ9189-21D2231Mod6/ao0") -> ()  [unwired: 6 in, 2 out]
                      }
                    }
                    frame #2 {
                      # "Max Voltage"
                      n164 = call "OnDemand_VoltageOutput.vi"("Channel Array"=dbl[] [5.067], "minimum voltage"=0.0, "maximum voltage"=5.067, "physical channels"="cDAQ9189-21D2231Mod6/ao0") -> ()  [unwired: 6 in, 2 out]
                      n165 = Wait (ms)(milliseconds to wait=u32 4000) -> ()  [unwired: 1 out]
                    }
                    frame #3 {
                      w279 = 6
                      n166 = for {
                        N: w279 -> [_]
                        shift-right: [w280] -> w277
                        shift-left: w278 -> [w286]
                        tunnel: w279 -> [_]
                        # "Max Voltage"
                        # "Until it reaches 2.067"
                        # "Reduce in steps of 0.5"
                        n167 = Subtract(x=w286, y=0.5) -> (x-y=w280:dbl[])
                        n168 = local write "Steps on Servo"(w280) -> ()
                        n169 = Wait (ms)(milliseconds to wait=u32 500) -> ()  [unwired: 1 out]
                        n170 = call "OnDemand_VoltageOutput.vi"("Channel Array"=w280, "minimum voltage"=0.0, "maximum voltage"=5.067, "physical channels"="cDAQ9189-21D2231Mod6/ao0") -> ()  [unwired: 6 in, 2 out]
                      }
                    }
                    frame #4 {
                      w289 = 6
                      n171 = for {
                        N: w289 -> [_]
                        shift-right: [w290] -> w287
                        shift-left: w288 -> [w296]
                        tunnel: w289 -> [_]
                        # "Max Voltage"
                        # "Until it reaches 2.067"
                        # "Increase in steps of 0.5"
                        n172 = Add(x=w296, y=0.5) -> (x+y=w290:dbl[])
                        n173 = local write "Steps on Servo"(w290) -> ()
                        n174 = Wait (ms)(milliseconds to wait=u32 500) -> ()  [unwired: 1 out]
                        n175 = call "OnDemand_VoltageOutput.vi"("Channel Array"=w290, "minimum voltage"=0.0, "maximum voltage"=5.067, "physical channels"="cDAQ9189-21D2231Mod6/ao0") -> ()  [unwired: 6 in, 2 out]
                      }
                    }
                    frame #5 {
                      w299 = 6
                      n176 = for {
                        N: w299 -> [_]
                        shift-right: [w300] -> w298
                        shift-left: w297 -> [w306]
                        tunnel: w299 -> [_]
                        # "Max Voltage"
                        # "Until it reaches 2.067"
                        # "Reduce in steps of 0.5"
                        n177 = Subtract(x=w306, y=0.5) -> (x-y=w300:dbl[])
                        n178 = local write "Steps on Servo"(w300) -> ()
                        n179 = Wait (ms)(milliseconds to wait=u32 500) -> ()  [unwired: 1 out]
                        n180 = call "OnDemand_VoltageOutput.vi"("Channel Array"=w300, "minimum voltage"=0.0, "maximum voltage"=5.067, "physical channels"="cDAQ9189-21D2231Mod6/ao0") -> ()  [unwired: 6 in, 2 out]
                      }
                    }
                    frame #6 {
                      n181 = for {
                        N: 6 -> [_]
                        shift-right: [w310] -> w307
                        shift-left: w308 -> [w316]
                        # "Max Voltage"
                        # "Until it reaches 2.067"
                        # "Increase in steps of 0.5"
                        n182 = Add(x=w316, y=0.5) -> (x+y=w310:dbl[])
                        n183 = local write "Steps on Servo"(w310) -> ()
                        n184 = Wait (ms)(milliseconds to wait=u32 500) -> ()  [unwired: 1 out]
                        n185 = call "OnDemand_VoltageOutput.vi"("Channel Array"=w310, "minimum voltage"=0.0, "maximum voltage"=5.067, "physical channels"="cDAQ9189-21D2231Mod6/ao0") -> ()  [unwired: 6 in, 2 out]
                      }
                    }
                    frame #7 {
                      w318 = 6
                      n186 = for {
                        N: w318 -> [_]
                        shift-right: [w319] -> _
                        shift-left: w317 -> [w325]
                        tunnel: w318 -> [_]
                        # "Max Voltage"
                        # "Until it reaches 2.067"
                        # "reduce in steps of 0.5"
                        n187 = Subtract(x=w325, y=0.5) -> (x-y=w319:dbl[])
                        n188 = local write "Steps on Servo"(w319) -> ()
                        n189 = Wait (ms)(milliseconds to wait=u32 500) -> ()  [unwired: 1 out]
                        n190 = call "OnDemand_VoltageOutput.vi"("Channel Array"=w319, "minimum voltage"=0.0, "maximum voltage"=5.067, "physical channels"="cDAQ9189-21D2231Mod6/ao0") -> ()  [unwired: 6 in, 2 out]
                      }
                    }
                    frame #8 {
                      w326 = dbl[] [0.0]
                      # "Reset to 0"
                      # "Max Voltage"
                      n191 = call "OnDemand_VoltageOutput.vi"("Channel Array"=w326, "minimum voltage"=0.0, "maximum voltage"=5.0, "physical channels"="cDAQ9189-21D2231Mod6/ao0") -> ()  [unwired: 6 in, 2 out]
                      n192 = local write "Steps on Servo"(w326) -> ()
                    }
                  }
                  n193 = while {
                    stop <- w254 stop-if-true
                    n194 = call "Elapsed Time2"() -> ("Elapsed Time (s)"=w252:dbl)  [unwired: 12 in, 7 out]
                    "Elapsed Time (s) 2" <- w252
                    n195 = global read "STOP_GLOBAL.vi" "ALL STOP"() -> (w254:bool)
                    n196 = Greater?(x=w252, y=3.0 ("x")) -> (0:→"HAS 3 SECONDS PASSED?":bool)
                  }
                }
              }
            }
            frame "Do nothing" {
            }
          }
          n197 = call <vilib>:"High Resolution Relative Seconds.vi"() -> ("relative seconds"=w66:dbl)
          n198 = while {
            tunnel: "Types of Testing" -> [w369]
            tunnel: [w403] -> w79 mode=indexing
            shift-right: [w396] -> w59
            shift-left: w63 -> [w398]
            shift-right: [w374] -> w60
            shift-left: w64 -> [w397]
            tunnel: [w383] -> w80 mode=indexing
            tunnel: [w381] -> w76 mode=indexing
            tunnel: [w380] -> w81 mode=indexing
            tunnel: [w379] -> w82 mode=indexing
            tunnel: [w375] -> w68 mode=indexing
            tunnel: [w359] -> w75 mode=indexing
            tunnel: [w382] -> w74 mode=indexing
            tunnel: w66 -> [w362]
            tunnel: w65 -> [_]
            tunnel: w61 -> [w358]
            stop <- w354 stop-if-true
            w342 = 110.0 ("x")
            w401 = 10.0  # timeout (s)
            # "Add SetPoint History\nAdd Gain history to data"
            # "First Test:\n2.1\n70\n3.566\nSecond:\n2.1\n80\n3.566\nThird:\n3.1\n60\n3.566\nFourth:\n10.1\n70\n3.566"
            # "Supply\nSecond Transducer\nFlow\nTemp\nOutput Voltage"
            # "4 NI 9219 Channels"
            # "Data Collection"
            n199 = call <vilib>:"High Resolution Relative Seconds.vi"() -> ("relative seconds"=w363:dbl)
            n200 = Subtract(x=w363, y=w362) -> (x-y=w360:dbl)
            n201 = Subtract(x=w360, y=0.0) -> (x-y=w359:dbl)
            "Entire Runtime" <- w359
            n202 = call-poly <vilib>:"DAQmx Read.vi"("task/channels in"=w397, "number of samples per channel"=-1, "timeout"=w401, "error in"=w398) -> ("task out"=w374:refnum<k21>, "data"=w399:waveform(dbl)[], "error out"=w396:errorcluster)  [unwired: 9 in]
            n203 = local read "PID gains out"() -> (w353:T3)
            n204 = local read "Actual Clock Rate"() -> (w365:dbl)
            n205 = global read "STOP_GLOBAL.vi" "ALL STOP"() -> (w400:bool)
            n206 = Split Signals(w399) -> (w345:dynamicdata, w346:dynamicdata, w356:dynamicdata, w395:dynamicdata, w355:dynamicdata, w394:dynamicdata, w343:dynamicdata, w344:dynamicdata)  [unwired: 15 in, 7 out]
            n207 = Unbundle By Name(w396) -> ("status"=w402:bool)
            n208 = Unbundle By Name(w353) -> ("proportional gain (Kc)"=w349:dbl, "integral time (Ti, min)"=w350:dbl, "derivative time (Td, min)"=w351:dbl)
            n209 = Divide(x=1.0, y=w365) -> (x/y=w364:dbl)
            n210 = local read "SP"() -> (w352:dbl)
            n211 = Or(x=w402, y=w400) -> (x .or. y?=w354:bool)
            n212 = Multiply(x=1000.0, y=w364) -> (x*y=w357:dbl)
            n213 = Wait Until Next ms Multiple(millisecond multiple=w357) -> ()  [unwired: 1 out]
            n214 = Merge Signals(w356, w395, w355, w394, w343, w344, w345, w346) -> (w393:dynamicdata)
            n215 = call "Convert to Dynamic Data2"("Double"=w349) -> ("Dynamic Data Type"=w337:dynamicdata)  [unwired: 3 in]
            n216 = call "Convert to Dynamic Data3"("Double"=w350) -> ("Dynamic Data Type"=w338:dynamicdata)  [unwired: 3 in]
            n217 = call "Convert to Dynamic Data4"("Double"=w351) -> ("Dynamic Data Type"=w339:dynamicdata)  [unwired: 3 in]
            n218 = call "Convert to Dynamic Data"("Double"=w352) -> ("Dynamic Data Type"=w340:dynamicdata)  [unwired: 3 in]
            n219 = call "Filter3"("Signal"=w393) -> ("Filtered Signal"=w391:dynamicdata)  [unwired: 9 in, 1 out]
            n220 = Split Signals(w391) -> (w373:dynamicdata, w372:dynamicdata, w371:dynamicdata, w370:dynamicdata, w334:dynamicdata, w332:dynamicdata, w336:dynamicdata, w335:dynamicdata)  [unwired: 8 in]
            n221 = local write "Temperature"(w335) -> ()
            n222 = Merge Signals(w373, w372, w370, w335, w332, w337, w338, w339, w340) -> (w348:dynamicdata)
            n223 = Multiply(x=w332, y=18.0) -> (x*y=w331:dynamicdata)
            n224 = local write "Voltage Output"(w331) -> ()
            n225 = Multiply(x=w342, y=w373) -> (x*y=w347:dynamicdata)
            n226 = Multiply(x=w342, y=w372) -> (x*y=w388:dynamicdata)
            n227 = Multiply(x=w342, y=w371) -> (x*y=w387:dynamicdata)
            n228 = Multiply(x=200.0, y=w370) -> (x*y=w385:dynamicdata)
            n229 = Multiply(x=w342, y=w334) -> (x*y=w341:dynamicdata)
            n230 = Merge Signals(w373, w372, w371, w370, w334, w336, w335, w332, w337, w338, w339, w340) -> (w368:dynamicdata)
            n231 = call "Convert from Dynamic Data11"("Dynamic Data Type"=w388) -> ("Array"=w389:dbl[])  [unwired: 3 in]
            n232 = call "Convert from Dynamic Data8"("Dynamic Data Type"=w347) -> ("Array"=w390:dbl[])  [unwired: 3 in]
            n233 = call "Convert from Dynamic Data12"("Dynamic Data Type"=w387) -> ("Array"=w386:dbl[])  [unwired: 3 in]
            n234 = call "Convert from Dynamic Data13"("Dynamic Data Type"=w385) -> ("Array"=w384:dbl[])  [unwired: 3 in]
            n235 = local write "Inlet Pressure"(w341) -> ()
            n236 = call-poly <vilib>:"Mean.vi"("X"=w390) -> ("mean"=w383:dbl)  [unwired: 1 out]
            n237 = call-poly <vilib>:"Mean.vi"("X"=w389) -> ("mean"=w382:dbl)  [unwired: 1 out]
            n238 = call-poly <vilib>:"Mean.vi"("X"=w386) -> ("mean"=w381:dbl)  [unwired: 1 out]
            n239 = call-poly <vilib>:"Mean.vi"("X"=w384) -> ("mean"=w380:dbl)  [unwired: 1 out]
            n240 = case shown="\"Test Firing\", Default" w369 {
              tunnel: w348 -> [_ w438]
              tunnel: w368 -> [w417 _]
              tunnel: w358 -> [w412 w429]
              frame "Test Firing", Default {
                n241 = Build Array("Supply Pressure", "Second Pressure Transducer", "Chamber Pressure", "Volumetric Flow", "Inlet Pressure", "Thrust", "Temperature", "Voltage Out" ("element"), "Kc" ("element"), "Ti" ("element"), "Td" ("element"), "Setpoint" ("element")) -> (w415:string[])
                n242 = call "RenameDynamicSignals.vi"("New Signal Names"=w415, "Dynamic Data In"=w417) -> ("error out"=w413:errorcluster, "Dynamic Data Out"=w414:dynamicdata)  [unwired: 2 in]
                n243 = call "Write To Measurement File3"("Signals"=w414, "Enable"="Collect Data?", "error in (no error)"=w413, "Filename"=w412) -> ("Filename Out"=→"Filename Out":path, "Saving Data"=→"Saving Data":bool, "error out"=→"error out 3":errorcluster)  [unwired: 13 in]
              }
              frame "Cold Flow Rig" {
                n244 = Build Array("Supply Pressure", "Second Pressure Transducer", "Volumetric Flow", "Temperature", "Voltage Out" ("element"), "Kc" ("element"), "Ti" ("element"), "Td" ("element"), "Setpoint" ("element")) -> (w432:string[])
                n245 = call "RenameDynamicSignals.vi"("New Signal Names"=w432, "Dynamic Data In"=w438) -> ("error out"=w430:errorcluster, "Dynamic Data Out"=w431:dynamicdata)  [unwired: 2 in]
                n246 = call "Write To Measurement File4"("Signals"=w431, "Enable"="Collect Data? 2", "error in (no error)"=w430, "Filename"=w429) -> ("Filename Out"=→"Filename Out":path, "Saving Data"=→"Saving Data":bool)  [unwired: 13 in, 1 out]
              }
            }
            n247 = local write "Supply Pressure PSI"(w347) -> ()
            n248 = local write "Second Pressure Transducer"(w388) -> ()
            n249 = local write "Thrust lb"(w336) -> ()
            n250 = local write "Chamber Pressure PSI"(w387) -> ()
            n251 = local write "Vol Flow L/min"(w385) -> ()
            n252 = call "Convert from Dynamic Data3"("Dynamic Data Type"=w335) -> ("Array"=w377:dbl[])  [unwired: 3 in]
            n253 = call "Convert from Dynamic Data4"("Dynamic Data Type"=w331) -> ("Array"=w376:dbl[])  [unwired: 3 in]
            n254 = call "Convert from Dynamic Data"("Dynamic Data Type"=w336) -> ("Array"=w378:dbl[])  [unwired: 3 in]
            n255 = call-poly <vilib>:"Mean.vi"("X"=w376) -> ("mean"=w375:dbl)  [unwired: 1 out]
            n256 = call-poly <vilib>:"Mean.vi"("X"=w378) -> ("mean"=w403:dbl)  [unwired: 1 out]
            n257 = call-poly <vilib>:"Mean.vi"("X"=w377) -> ("mean"=w379:dbl)  [unwired: 1 out]
          }
          n258 = call <vilib>:"DAQmx Stop Task.vi"("task/channels in"=w60, "error in"=w59) -> ("task out"=w57:refnum<k21>, "error out"=w58:errorcluster)  [unwired: 12 in]
          n259 = call <vilib>:"DAQmx Clear Task.vi"("task in"=w57, "error in"=w58) -> ("error out"=w56:errorcluster)  [unwired: 13 in]
          "error out 2" <- w56
          n260 = Bundle(w75, w74) -> (w73:cluster{dbl[], dbl[]})  [unwired: 1 in]
          "Second Pressure Transducer" <- w73
          n261 = Bundle(w75, w76) -> (w72:cluster{dbl[], dbl[]})  [unwired: 1 in]
          "Chamber Pressure" <- w72
          n262 = Bundle(w75, w80) -> (w78:cluster{dbl[], dbl[]})  [unwired: 1 in]
          "Supply Pressure" <- w78
          n263 = Bundle(w75, w81) -> (w71:cluster{dbl[], dbl[]})  [unwired: 1 in]
          "MassFlow" <- w71
          n264 = Bundle(w75, w79) -> (w70:cluster{dbl[], dbl[]})  [unwired: 1 in]
          "Thrust" <- w70
          n265 = Bundle(w75, w82) -> (w69:cluster{dbl[], dbl[]})  [unwired: 1 in]
          "Temperature" <- w69
          n266 = Bundle(w75, w68) -> (→"Servo Voltage Output":cluster{dbl[], dbl[]})  [unwired: 1 in]
          n267 = call <vilib>:"Simple Error Handler.vi"("error in (no error)"=w56) -> ()  [unwired: 4 in, 5 out]
          n268 = Build Array(w78, w73, w72, w71, w70, w69) -> (→"All Channel Graph":cluster{dbl[], dbl[]}[])
        }
      }
    }
  }
